vi "_sp3.vi"(5 "sp_data":T3={"total data num(1-3)"=2, "file_name"="", "SAVE OFF/ON"=TRUE, "ATT1"=5.0, "ATT2"=7.0, "SNAdatafile ATT1"=path "C:/Documents and Settings/?澤佳?/デスクトップ/MIX99/100217_ifbox/5dB.prn", "SNAdatafile ATT2"=path "C:/Documents and Settings/?澤佳?/デスクトップ/MIX99/100217_ifbox/7dB.prn", "ATTcal"=TRUE, "SP_set"={"start(GHz)"=3.5, "stop(GHz) "=12.5, "BW(MHz)"=8.0, "VBW(Hz)"=30.0, "ref(dBm)"=-45.0, "log(dB)"=1.0, "AVEG"=1, "AVEG ON/OFF"=FALSE, "Auto Align ON/OFF"=FALSE, "GPIB"="18", "point"=801}, "HOT/COLD"=0} {"HOT/COLD" items=["Manual", "Motor auto", "SIS V", "P0/P1", "sinlge data"]}, 6 "Control":T2={"GPIB_ATT"="28", "6501Dev#"=1, "GPIB_SP"="18", "GPIB_PM"="13", "GPIB_DSA"="11", "GPIB_DMM (TPD)"="23", "GPIB_MPI"="2", "mortor設定"=[{"Axis"=0, "ID"=0, "HIspeed"=200.0, "LOspeed"=100.0, "ACCEL(ms)"=100.0, "Sratio"=50.0, "フリーラン\n"=TRUE, "文字列"="DSB HOT/COLD"}, {"Axis"=1, "ID"=0, "HIspeed"=4.0, "LOspeed"=4.0, "ACCEL(ms)"=100.0, "Sratio"=50.0, "フリーラン\n"=TRUE, "文字列"="SubMM Att"}], "DATAパス"=path "Z:/band10/Labview_ALMA/MIX95/test", "DBパス "=path "Z:/band10/Labview_ALMA/MIX95/test", "comment"="P1_Tmin", "ColdCarts"="003601", "Th"=295.0, "Tc"=77.0, "Set_SIS_volt"=2.1, "Offset"=0.0, "control"=0, "FreqLO"=800.0, "Set_Mag_Cur"=800.0, "MPI offset(mm)"=22.99, "HOT/COLD"=0} {"HOT/COLD" items=["DSB", "SBR", "GainComp"]; "control" items=["CLOSE LOOP", "OPEN LOOP", "Not Control"]}, 7 "Bias_LO_equip":T1={"Node address"=19, "CAN Interface"="CAN0", "Cartridge band"=10, "Slave Node in"={"Address"=19, "Serial Number"=[16, 71, 55, 76, 1, 8, 0, -15]}, "ObjHandle out"=170917952, "POL"=1, "sb"=1, "GPIB_SM (SIS S,V)"="24", "GPIB_DMM (SIS I)"="22", "GPIB_SM (MAG I) "="25", "GPIB_SG(LO)"="19", "GPIB_PW (PAMP) "="6", "GPIB_TMP1(8ch)"="12", "GPIB_TMP2(2ch)  "="13", "WCA_avg"=10, "Rsen"=10.0, "BiasModule"=1, "LOModule "=5, "WCA_LO_FREQ_SET"={"YTO Low freq. [GHz]"=14.42, "YTO High freq. [GHz]"=17.7, "Kvco"=1, "Lock Pol."=0, "SET LO FREQ"=97.111115, "Multiplier"=6.0, "YTO (HEX)"=2196, "YTO ( FREQ)"=16.178946, "NULL PLL INTEGRATOR"=FALSE}, "Res for"=0} {"Res for" items=["none", "series res", "parallel res"]; "WCA_LO_FREQ_SET"."YTO ( FREQ)" min=25 max=150 step=0.0001 format="%.3f"; "WCA_LO_FREQ_SET"."Multiplier" min=3 max=6 step=3; "WCA_LO_FREQ_SET"."SET LO FREQ" min=25 max=150 step=0.0001 format="%.3f"; "WCA_LO_FREQ_SET"."Lock Pol." items=["Lower", "Upper"]; "WCA_LO_FREQ_SET"."Kvco" items=["7.5MHz/V", "15MHz/V"]; "WCA_LO_FREQ_SET"."YTO High freq. [GHz]" format="%.3f"; "WCA_LO_FREQ_SET"."YTO Low freq. [GHz]" format="%.3f"; "LOModule" items=["Manual Gunn+PAMP"=0, "PLL GUNN+PAMP"=5, "B10Lab LO"=1, "WCA LO"=2, ""=3, "YIG発信器"=4, "none"=99]; "BiasModule" items=["B10Lab Bias"=0, "WCA BiasModule"=1, "none"=99]; "Slave Node in"."Serial Number" format="%.0x"; "Slave Node in"."Address" format="%.0x"; "Cartridge band" max=10 step=1; "Node address" format="%.0x"}) -> ()   [LabVIEW 2017]
uses:
  <vilib>/Utility/file.llb/Read From Spreadsheet File (DBL).vi
  <vilib>/express/express arith-compare/Formula/XNode/ExpressFormulaBlockNode.xnode
  <vilib>/gmath/NI_Gmath.lvlib
panel:
  in  "HOT/COLD AUTO":bool=TRUE
  in  "タブ制御器":enum32{"ページ 1", "ページ 2"}(tab)
  out "XYグラフ":cluster{dbl, dbl}[](graph)=[{3.5, -71.954}, {3.51125, -71.842}, {3.5225, -71.893}, {3.53375, -72.314}, {3.545, -72.393}, {3.55625, -71.859}, {3.5675, -71.184}, {3.57875, -69.995}, {3.59, -68.081}, {3.60125, -65.91}, {3.6125, -64.753}, {3.62375, -64.752}, {3.635, -65.026}, {3.64625, -65.45}, {3.6575, -64.906}, {3.66875, -63.764}, {3.68, -62.097}, {3.69125, -60.126}, {3.7025, -58.665}, {3.71375, -58.024}, {3.725, -57.93}, {3.73625, -57.927}, {3.7475, -57.979}, {3.75875, -57.611}, {3.77, -56.352}, {3.78125, -54.399}, {3.7925, -52.484}, {3.80375, -51.209}, {3.815, -50.629}, {3.82625, -50.38}, {3.8375, -50.206}, {3.84875, -50.084}, {3.86, -49.915}, {3.87125, -49.525}, {3.8825, -49.077}, {3.89375, -48.4}, {3.905, -47.812}, {3.91625, -47.508}, {3.9275, -47.326}, {3.93875, -47.27}, {3.95, -47.088}, {3.96125, -46.924}, {3.9725, -46.838}, {3.98375, -46.867}, {3.995, -46.862}, {4.00625, -46.788}, {4.0175, -46.715}, {4.02875, -46.722}, {4.04, -46.709}, {4.05125, -46.62}, {4.0625, -46.617}, {4.07375, -46.606}, {4.085, -46.621}, {4.09625, -46.532}, {4.1075, -46.451}, {4.11875, -46.457}, {4.13, -46.365}, {4.14125, -46.296}, {4.1525, -46.289}, {4.16375, -46.373}, {4.175, -46.372}, {4.18625, -46.286}, {4.1975, -46.224}, {4.20875, -46.246}, {4.22, -46.278}, {4.23125, -46.252}, {4.2425, -46.205}, {4.25375, -46.184}, {4.265, -46.167}, {4.27625, -46.168}, {4.2875, -46.147}, {4.29875, -46.094}, {4.31, -46.092}, {4.32125, -46.151}, {4.3325, -46.218}, {4.34375, -46.256}, {4.355, -46.233}, {4.36625, -46.182}, {4.3775, -46.22}, {4.38875, -46.223}, {4.4, -46.301}, {4.41125, -46.386}, {4.4225, -46.511}, {4.43375, -46.483}, {4.445, -46.367}, {4.45625, -46.279}, {4.4675, -46.251}, {4.47875, -46.241}, {4.49, -46.238}, {4.50125, -46.231}, {4.5125, -46.219}, {4.52375, -46.147}, {4.535, -46.095}, {4.54625, -46.112}, {4.5575, -46.151}, {4.56875, -46.067}, {4.58, -46.01}, {4.59125, -45.981}, {4.6025, -46.006}, {4.61375, -46.047}, {4.625, -46.085}, {4.63625, -46.099}, {4.6475, -46.104}, {4.65875, -46.087}, {4.67, -46.069}, {4.68125, -46.087}, {4.6925, -46.163}, {4.70375, -46.198}, {4.715, -46.218}, {4.72625, -46.189}, {4.7375, -46.188}, {4.74875, -46.232}, {4.76, -46.248}, {4.77125, -46.379}, {4.7825, -46.515}, {4.79375, -46.613}, {4.805, -46.671}, {4.81625, -46.713}, {4.8275, -46.773}, {4.83875, -46.799}, {4.85, -46.868}, {4.86125, -46.939}, {4.8725, -46.989}, {4.88375, -47.123}, {4.895, -47.176}, {4.90625, -47.133}, {4.9175, -47.123}, {4.92875, -47.067}, {4.94, -47.068}, {4.95125, -47.108}, {4.9625, -47.197}, {4.97375, -47.251}, {4.985, -47.163}, {4.99625, -47.078}, {5.0075, -47.106}, {5.01875, -47.261}, {5.03, -47.236}, {5.04125, -47.088}, {5.0525, -47.01}, {5.06375, -47.036}, {5.075, -47.175}, {5.08625, -47.19}, {5.0975, -47.053}, {5.10875, -46.876}, {5.12, -46.702}, {5.13125, -46.717}, {5.1425, -46.72}, {5.15375, -46.718}, {5.165, -46.753}, {5.17625, -46.853}, {5.1875, -46.973}, {5.19875, -47.25}, {5.21, -47.402}, {5.22125, -47.146}, {5.2325, -47.002}, {5.24375, -46.974}, {5.255, -46.975}, {5.26625, -47.063}, {5.2775, -47.135}, {5.28875, -47.209}, {5.3, -47.278}, {5.31125, -47.27}, {5.3225, -47.272}, {5.33375, -47.282}, {5.345, -47.266}, {5.35625, -47.26}, {5.3675, -47.263}, {5.37875, -47.404}, {5.39, -47.446}, {5.40125, -47.366}, {5.4125, -47.323}, {5.42375, -47.361}, {5.435, -47.465}, {5.44625, -47.472}, {5.4575, -47.381}, {5.46875, -47.304}, {5.48, -47.288}, {5.49125, -47.333}, {5.5025, -47.467}, {5.51375, -47.458}, {5.525, -47.323}, {5.53625, -47.264}, {5.5475, -47.27}, {5.55875, -47.335}, {5.57, -47.249}, {5.58125, -47.105}, {5.5925, -47.044}, {5.60375, -47.03}, {5.615, -47.109}, {5.62625, -47.09}, {5.6375, -46.967}, {5.64875, -46.926}, {5.66, -46.942}, {5.67125, -47.103}, {5.6825, -47.225}, {5.69375, -47.112}, {5.705, -46.983}, {5.71625, -46.925}, {5.7275, -46.934}, {5.73875, -46.981}, {5.75, -47.024}, {5.76125, -47.033}, {5.7725, -47.114}, {5.78375, -47.206}, {5.795, -47.097}, {5.80625, -47.025}, {5.8175, -46.985}, {5.82875, -46.993}, {5.84, -47.125}, {5.85125, -47.259}, {5.8625, -47.344}, {5.87375, -47.276}, {5.885, -47.267}, {5.89625, -47.347}, {5.9075, -47.507}, {5.91875, -47.473}, {5.93, -47.345}, {5.94125, -47.275}, {5.9525, -47.288}, {5.96375, -47.47}, {5.975, -47.534}, {5.98625, -47.542}, {5.9975, -47.499}, {6.00875, -47.515}, {6.02, -47.607}, {6.03125, -47.748}, {6.0425, -47.648}, {6.05375, -47.578}, {6.065, -47.508}, {6.07625, -47.476}, {6.0875, -47.547}, {6.09875, -47.594}, {6.11, -47.534}, {6.12125, -47.453}, {6.1325, -47.326}, {6.14375, -47.297}, {6.155, -47.288}, {6.16625, -47.203}, {6.1775, -47.151}, {6.18875, -47.076}, {6.2, -47.058}, {6.21125, -46.98}, {6.2225, -46.939}, {6.23375, -46.893}, {6.245, -46.988}, {6.25625, -47.016}, {6.2675, -46.998}, {6.27875, -46.991}, {6.29, -46.946}, {6.30125, -46.945}, {6.3125, -47.01}, {6.32375, -47.183}, {6.335, -47.328}, {6.34625, -47.41}, {6.3575, -47.315}, {6.36875, -47.32}, {6.38, -47.479}, {6.39125, -47.474}, {6.4025, -47.433}, {6.41375, -47.457}, {6.425, -47.6}, {6.43625, -47.833}, {6.4475, -47.912}, {6.45875, -47.849}, {6.47, -47.844}, {6.48125, -47.87}, {6.4925, -47.94}, {6.50375, -47.984}, {6.515, -47.973}, {6.52625, -47.994}, {6.5375, -48.059}, {6.54875, -48.054}, {6.56, -48.117}, {6.57125, -48.268}, {6.5825, -48.212}, {6.59375, -48.119}, {6.605, -48.06}, {6.61625, -48.022}, {6.6275, -47.989}, {6.63875, -47.931}, {6.65, -47.939}, {6.66125, -47.992}, {6.6725, -47.963}, {6.68375, -47.893}, {6.695, -47.572}, {6.70625, -47.495}, {6.7175, -47.442}, {6.72875, -47.459}, {6.74, -47.385}, {6.75125, -47.361}, {6.7625, -47.311}, {6.77375, -47.208}, {6.785, -47.211}, {6.79625, -47.241}, {6.8075, -47.208}, {6.81875, -47.2}, {6.83, -47.225}, {6.84125, -47.271}, {6.8525, -47.437}, {6.86375, -47.61}, {6.875, -47.614}, {6.88625, -47.644}, {6.8975, -47.731}, {6.90875, -47.757}, {6.92, -47.789}, {6.93125, -47.736}, {6.9425, -47.737}, {6.95375, -47.619}, {6.965, -47.373}, {6.97625, -47.303}, {6.9875, -47.287}, {6.99875, -47.276}, {7.01, -47.34}, {7.02125, -47.491}, {7.0325, -47.621}, {7.04375, -47.843}, {7.055, -47.873}, {7.06625, -47.802}, {7.0775, -47.764}, {7.08875, -47.787}, {7.1, -47.793}, {7.11125, -47.733}, {7.1225, -47.469}, {7.13375, -47.271}, {7.145, -47.145}, {7.15625, -47.097}, {7.1675, -47.072}, {7.17875, -47.143}, {7.19, -47.234}, {7.20125, -47.288}, {7.2125, -47.346}, {7.22375, -47.39}, {7.235, -47.533}, {7.24625, -47.358}, {7.2575, -47.209}, {7.26875, -47.056}, {7.28, -46.933}, {7.29125, -46.892}, {7.3025, -46.642}, {7.31375, -46.487}, {7.325, -46.441}, {7.33625, -46.415}, {7.3475, -46.343}, {7.35875, -46.318}, {7.37, -46.302}, {7.38125, -46.537}, {7.3925, -46.847}, {7.40375, -46.854}, {7.415, -46.841}, {7.42625, -46.902}, {7.4375, -47.021}, {7.44875, -47.161}, {7.46, -47.435}, {7.47125, -47.781}, {7.4825, -47.531}, {7.49375, -47.405}, {7.505, -47.501}, {7.51625, -47.665}, {7.5275, -47.625}, {7.53875, -47.527}, {7.55, -47.453}, {7.56125, -47.592}, {7.5725, -47.723}, {7.58375, -47.43}, {7.595, -47.291}, {7.60625, -47.215}, {7.6175, -47.141}, {7.62875, -47.18}, {7.64, -47.309}, {7.65125, -47.525}, {7.6625, -47.415}, {7.67375, -47.178}, {7.685, -47.025}, {7.69625, -47.063}, {7.7075, -47.163}, {7.71875, -47.172}, {7.73, -47.341}, {7.74125, -47.497}, {7.7525, -47.465}, {7.76375, -47.238}, {7.775, -47.125}, {7.78625, -47.038}, {7.7975, -47.035}, {7.80875, -46.956}, {7.82, -46.887}, {7.83125, -46.691}, {7.8425, -46.535}, {7.85375, -46.453}, {7.865, -46.413}, {7.87625, -46.469}, {7.8875, -46.594}, {7.89875, -46.746}, {7.91, -46.859}, {7.92125, -47.036}, {7.9325, -47.214}, {7.94375, -47.294}, {7.955, -47.195}, {7.96625, -47.173}, {7.9775, -47.245}, {7.98875, -47.48}, {8.0, -47.468}, {8.01125, -47.138}, {8.0225, -46.85}, {8.03375, -46.737}, {8.045, -46.672}, {8.05625, -46.651}, {8.0675, -46.728}, {8.07875, -46.881}, {8.09, -47.039}, {8.10125, -47.059}, {8.1125, -47.027}, {8.12375, -47.041}, {8.135, -47.131}, {8.14625, -47.264}, {8.1575, -47.113}, {8.16875, -46.901}, {8.18, -46.669}, {8.19125, -46.499}, {8.2025, -46.442}, {8.21375, -46.451}, {8.225, -46.571}, {8.23625, -46.545}, {8.2475, -46.48}, {8.25875, -46.493}, {8.27, -46.494}, {8.28125, -46.454}, {8.2925, -46.493}, {8.30375, -46.766}, {8.315, -46.888}, {8.32625, -46.929}, {8.3375, -46.778}, {8.34875, -46.53}, {8.36, -46.506}, {8.37125, -46.633}, {8.3825, -46.912}, {8.39375, -47.149}, {8.405, -47.02}, {8.41625, -47.011}, {8.4275, -47.041}, {8.43875, -46.9}, {8.45, -46.848}, {8.46125, -46.941}, {8.4725, -47.126}, {8.48375, -47.289}, {8.495, -47.597}, {8.50625, -47.67}, {8.5175, -47.639}, {8.52875, -47.57}, {8.54, -47.643}, {8.55125, -47.999}, {8.5625, -48.482}, {8.57375, -48.445}, {8.585, -48.386}, {8.59625, -48.295}, {8.6075, -48.254}, {8.61875, -48.367}, {8.63, -48.398}, {8.64125, -48.483}, {8.6525, -48.862}, {8.66375, -48.682}, {8.675, -48.434}, {8.68625, -48.456}, {8.6975, -48.453}, {8.70875, -48.478}, {8.72, -48.475}, {8.73125, -48.559}, {8.7425, -48.753}, {8.75375, -48.633}, {8.765, -48.485}, {8.77625, -48.4}, {8.7875, -48.376}, {8.79875, -48.436}, {8.81, -48.56}, {8.82125, -48.668}, {8.8325, -48.756}, {8.84375, -48.81}, {8.855, -48.76}, {8.86625, -48.771}, {8.8775, -48.915}, {8.88875, -48.911}, {8.9, -48.871}, {8.91125, -48.87}, {8.9225, -48.91}, {8.93375, -48.989}, {8.945, -48.962}, {8.95625, -49.024}, {8.9675, -49.068}, {8.97875, -49.178}, {8.99, -49.307}, {9.00125, -49.438}, {9.0125, -49.343}, {9.02375, -49.306}, {9.035, -49.359}, {9.04625, -49.633}, {9.0575, -49.932}, {9.06875, -49.957}, {9.08, -49.924}, {9.09125, -49.955}, {9.1025, -50.016}, {9.11375, -50.034}, {9.125, -50.167}, {9.13625, -50.212}, {9.1475, -50.193}, {9.15875, -50.317}, {9.17, -50.568}, {9.18125, -50.694}, {9.1925, -50.942}, {9.20375, -50.843}, {9.215, -50.756}, {9.22625, -50.768}, {9.2375, -50.987}, {9.24875, -50.892}, {9.26, -50.838}, {9.27125, -50.868}, {9.2825, -50.777}, {9.29375, -50.499}, {9.305, -50.274}, {9.31625, -50.154}, {9.3275, -50.137}, {9.33875, -50.183}, {9.35, -50.199}, {9.36125, -50.095}, {9.3725, -50.004}, {9.38375, -49.996}, {9.395, -50.088}, {9.40625, -50.265}, {9.4175, -50.351}, {9.42875, -50.126}, {9.44, -49.893}, {9.45125, -49.901}, {9.4625, -49.87}, {9.47375, -49.79}, {9.485, -49.584}, {9.49625, -49.419}, {9.5075, -49.492}, {9.51875, -49.658}, {9.53, -49.972}, {9.54125, -50.161}, {9.5525, -50.298}, {9.56375, -50.405}, {9.575, -50.455}, {9.58625, -50.619}, {9.5975, -50.83}, {9.60875, -51.11}, {9.62, -51.061}, {9.63125, -51.029}, {9.6425, -51.011}, {9.65375, -51.013}, {9.665, -51.056}, {9.67625, -51.14}, {9.6875, -51.281}, {9.69875, -51.296}, {9.71, -51.39}, {9.72125, -51.515}, {9.7325, -51.685}, {9.74375, -51.81}, {9.755, -51.972}, {9.76625, -52.069}, {9.7775, -52.084}, {9.78875, -52.083}, {9.8, -52.012}, {9.81125, -52.005}, {9.8225, -51.769}, {9.83375, -51.503}, {9.845, -51.371}, {9.85625, -51.273}, {9.8675, -51.381}, {9.87875, -51.376}, {9.89, -51.116}, {9.90125, -50.863}, {9.9125, -50.64}, {9.92375, -50.582}, {9.935, -50.576}, {9.94625, -50.736}, {9.9575, -50.904}, {9.96875, -50.964}, {9.98, -51.343}, {9.99125, -51.665}, {10.0025, -51.61}, {10.01375, -51.443}, {10.025, -51.439}, {10.03625, -51.317}, {10.0475, -51.287}, {10.05875, -51.528}, {10.07, -51.818}, {10.08125, -51.83}, {10.0925, -51.847}, {10.10375, -51.65}, {10.115, -51.395}, {10.12625, -51.146}, {10.1375, -51.112}, {10.14875, -51.144}, {10.16, -51.204}, {10.17125, -51.391}, {10.1825, -51.63}, {10.19375, -51.824}, {10.205, -51.848}, {10.21625, -51.941}, {10.2275, -52.093}, {10.23875, -52.046}, {10.25, -52.017}, {10.26125, -52.211}, {10.2725, -52.345}, {10.28375, -52.094}, {10.295, -51.887}, {10.30625, -51.816}, {10.3175, -51.905}, {10.32875, -52.242}, {10.34, -52.607}, {10.35125, -52.478}, {10.3625, -52.33}, {10.37375, -52.199}, {10.385, -52.036}, {10.39625, -52.019}, {10.4075, -52.159}, {10.41875, -52.303}, {10.43, -51.947}, {10.44125, -51.68}, {10.4525, -51.689}, {10.46375, -52.1}, {10.475, -52.598}, {10.48625, -52.325}, {10.4975, -52.164}, {10.50875, -52.263}, {10.52, -52.392}, {10.53125, -52.562}, {10.5425, -52.581}, {10.55375, -52.684}, {10.565, -52.683}, {10.57625, -52.908}, {10.5875, -53.461}, {10.59875, -54.026}, {10.61, -53.447}, {10.62125, -53.018}, {10.6325, -52.82}, {10.64375, -52.542}, {10.655, -52.227}, {10.66625, -51.967}, {10.6775, -51.823}, {10.68875, -51.83}, {10.7, -52.037}, {10.71125, -52.406}, {10.7225, -52.612}, {10.73375, -52.958}, {10.745, -53.193}, {10.75625, -53.38}, {10.7675, -53.503}, {10.77875, -53.482}, {10.79, -53.314}, {10.80125, -53.149}, {10.8125, -53.048}, {10.82375, -52.998}, {10.835, -53.048}, {10.84625, -53.039}, {10.8575, -53.25}, {10.86875, -53.51}, {10.88, -53.135}, {10.89125, -52.842}, {10.9025, -52.76}, {10.91375, -52.749}, {10.925, -53.082}, {10.93625, -53.424}, {10.9475, -53.489}, {10.95875, -53.431}, {10.97, -53.218}, {10.98125, -53.083}, {10.9925, -52.862}, {11.00375, -52.702}, {11.015, -52.589}, {11.02625, -52.395}, {11.0375, -52.351}, {11.04875, -52.493}, {11.06, -52.789}, {11.07125, -52.657}, {11.0825, -52.484}, {11.09375, -52.469}, {11.105, -52.515}, {11.11625, -52.733}, {11.1275, -52.718}, {11.13875, -52.712}, {11.15, -52.705}, {11.16125, -52.773}, {11.1725, -52.926}, {11.18375, -53.285}, {11.195, -53.63}, {11.20625, -53.688}, {11.2175, -53.507}, {11.22875, -53.483}, {11.24, -53.567}, {11.25125, -53.872}, {11.2625, -53.942}, {11.27375, -53.909}, {11.285, -53.962}, {11.29625, -54.009}, {11.3075, -54.13}, {11.31875, -54.282}, {11.33, -54.512}, {11.34125, -54.993}, {11.3525, -54.907}, {11.36375, -54.589}, {11.375, -54.365}, {11.38625, -54.0}, {11.3975, -53.84}, {11.40875, -53.788}, {11.42, -53.787}, {11.43125, -53.917}, {11.4425, -54.185}, {11.45375, -54.528}, {11.465, -54.871}, {11.47625, -54.573}, {11.4875, -54.388}, {11.49875, -54.433}, {11.51, -54.668}, {11.52125, -54.887}, {11.5325, -55.037}, {11.54375, -55.076}, {11.555, -55.133}, {11.56625, -54.956}, {11.5775, -54.649}, {11.58875, -54.536}, {11.6, -54.508}, {11.61125, -54.439}, {11.6225, -54.513}, {11.63375, -54.746}, {11.645, -55.053}, {11.65625, -55.34}, {11.6675, -55.542}, {11.67875, -55.519}, {11.69, -55.354}, {11.70125, -55.181}, {11.7125, -55.089}, {11.72375, -54.965}, {11.735, -54.856}, {11.74625, -54.901}, {11.7575, -55.157}, {11.76875, -55.323}, {11.78, -55.286}, {11.79125, -55.066}, {11.8025, -54.962}, {11.81375, -54.984}, {11.825, -55.109}, {11.83625, -55.261}, {11.8475, -55.068}, {11.85875, -54.862}, {11.87, -54.783}, {11.88125, -54.818}, {11.8925, -54.664}, {11.90375, -54.832}, {11.915, -54.974}, {11.92625, -55.083}, {11.9375, -55.33}, {11.94875, -55.714}, {11.96, -56.097}, {11.97125, -55.931}, {11.9825, -55.862}, {11.99375, -55.928}, {12.005, -56.047}, {12.01625, -55.985}, {12.0275, -55.847}, {12.03875, -56.034}, {12.05, -55.922}, {12.06125, -55.8}, {12.0725, -55.771}, {12.08375, -55.593}, {12.095, -55.6}, {12.10625, -55.918}, {12.1175, -56.305}, {12.12875, -56.413}, {12.14, -56.4}, {12.15125, -56.827}, {12.1625, -57.471}, {12.17375, -58.045}, {12.185, -57.987}, {12.19625, -57.899}, {12.2075, -57.938}, {12.21875, -57.8}, {12.23, -58.004}, {12.24125, -58.753}, {12.2525, -59.581}, {12.26375, -60.009}, {12.275, -59.706}, {12.28625, -59.607}, {12.2975, -59.689}, {12.30875, -60.204}, {12.32, -61.1}, {12.33125, -62.589}, {12.3425, -64.312}, {12.35375, -65.705}, {12.365, -66.003}, {12.37625, -65.213}, {12.3875, -64.672}, {12.39875, -64.666}, {12.41, -64.945}, {12.42125, -65.677}, {12.4325, -66.563}, {12.44375, -67.347}, {12.455, -67.766}, {12.46625, -67.937}, {12.4775, -68.115}, {12.48875, -68.108}, {12.5, -67.876}]
  out "XYグラフ 2":cluster{dbl, dbl}[](graph)=[{3.5, 262.8761923486348}, {3.51125, 265.3941119007726}, {3.5225, 261.20275301828303}, {3.53375, 254.61452613630323}, {3.545, 265.256944327723}, {3.55625, 256.71770445279355}, {3.5675, 253.29895702347693}, {3.57875, 255.931422963521}, {3.59, 257.1114683734254}, {3.60125, 255.75498871941952}, {3.6125, 250.5281702924347}, {3.62375, 240.4459191545401}, {3.635, 245.18716604138476}, {3.64625, 238.9567024993202}, {3.6575, 236.97953138656834}, {3.66875, 254.50165799946515}, {3.68, 242.07864861705457}, {3.69125, 244.50359101739548}, {3.7025, 224.949128515961}, {3.71375, 225.85065303629233}, {3.725, 228.89158214555707}, {3.73625, 229.3093007737749}, {3.7475, 228.17456602724567}, {3.75875, 231.41887343795008}, {3.77, 240.36727143390723}, {3.78125, 224.65040280568107}, {3.7925, 227.2627743063754}, {3.80375, 239.43391314174212}, {3.815, 247.8165740086698}, {3.82625, 245.15636147038293}, {3.8375, 240.82133483850794}, {3.84875, 244.21563567548085}, {3.86, 244.4827666625702}, {3.87125, 244.08831190861994}, {3.8825, 241.8090904197592}, {3.89375, 244.34243732142812}, {3.905, 244.67617340165324}, {3.91625, 242.69332978130743}, {3.9275, 240.47841129027896}, {3.93875, 235.47071382602226}, {3.95, 241.93528131929722}, {3.96125, 241.89546730654737}, {3.9725, 241.86385478544392}, {3.98375, 236.56768322757807}, {3.995, 238.7902448928445}, {4.00625, 247.50639151841088}, {4.0175, 245.57315502756728}, {4.02875, 241.90119061580842}, {4.04, 243.33931405889274}, {4.05125, 243.10170518604278}, {4.0625, 244.04149874278417}, {4.07375, 246.9641892769639}, {4.085, 238.61123449304475}, {4.09625, 242.9462880124439}, {4.1075, 244.5051542938281}, {4.11875, 244.12106797294564}, {4.13, 240.57466833749857}, {4.14125, 240.8274300472488}, {4.1525, 243.30389434626068}, {4.16375, 240.68284134010386}, {4.175, 239.34447201355923}, {4.18625, 245.05443426912723}, {4.1975, 245.682449223128}, {4.20875, 245.80306076988367}, {4.22, 248.0206300592133}, {4.23125, 242.02207084394269}, {4.2425, 246.9183927125329}, {4.25375, 243.05566615613813}, {4.265, 249.08045120777058}, {4.27625, 247.13970788273744}, {4.2875, 240.30192904146838}, {4.29875, 245.41878418214426}, {4.31, 241.7558889355493}, {4.32125, 241.31125347787935}, {4.3325, 243.2220561500085}, {4.34375, 231.30252460707732}, {4.355, 235.44495546231832}, {4.36625, 244.56412835893218}, {4.3775, 237.0241031165103}, {4.38875, 239.04193968622735}, {4.4, 236.43738406649962}, {4.41125, 236.94651077829408}, {4.4225, 234.76613596800598}, {4.43375, 236.369466168867}, {4.445, 236.8802182641571}, {4.45625, 239.50967040948262}, {4.4675, 237.3156198339352}, {4.47875, 233.35482141391896}, {4.49, 234.39853864941963}, {4.50125, 232.93326616359997}, {4.5125, 230.8352049801077}, {4.52375, 235.480258435589}, {4.535, 238.0804283666065}, {4.54625, 243.96822176961183}, {4.5575, 233.56300311786632}, {4.56875, 237.6484876135124}, {4.58, 237.07719132394985}, {4.59125, 240.06151036000696}, {4.6025, 239.16401930247414}, {4.61375, 240.853494620256}, {4.625, 237.24016928691904}, {4.63625, 237.0012418390217}, {4.6475, 236.19054957073072}, {4.65875, 232.79019526262627}, {4.67, 234.41802454613145}, {4.68125, 236.71013995490105}, {4.6925, 234.94960077269158}, {4.70375, 242.74225771843138}, {4.715, 230.69626423612328}, {4.72625, 237.99671249942847}, {4.7375, 243.19972698657756}, {4.74875, 241.78564535897496}, {4.76, 246.68989579012796}, {4.77125, 233.77252393131778}, {4.7825, 232.74807333114165}, {4.79375, 237.3375087150141}, {4.805, 236.843220223869}, {4.81625, 238.62876135740984}, {4.8275, 237.65852913341678}, {4.83875, 242.60928819707286}, {4.85, 236.5923218121674}, {4.86125, 233.1555591792413}, {4.8725, 248.21294191750152}, {4.88375, 238.63927518318636}, {4.895, 236.6411303958895}, {4.90625, 238.84550812970093}, {4.9175, 239.8289353237909}, {4.92875, 233.29071763362768}, {4.94, 232.47060195525304}, {4.95125, 233.54853283996468}, {4.9625, 232.80149118225611}, {4.97375, 234.11503048456947}, {4.985, 234.4759190982286}, {4.99625, 236.5417413984665}, {5.0075, 237.41562271675028}, {5.01875, 239.9997205474734}, {5.03, 238.58613987506754}, {5.04125, 232.48363592932222}, {5.0525, 235.53513669533723}, {5.06375, 234.33804621510708}, {5.075, 241.269198219873}, {5.08625, 234.02323477825186}, {5.0975, 242.29718074124258}, {5.10875, 236.02463840576507}, {5.12, 236.95944040804943}, {5.13125, 238.55613692219285}, {5.1425, 242.4470435889024}, {5.15375, 239.3502543997521}, {5.165, 238.91000188022844}, {5.17625, 239.31305101575524}, {5.1875, 237.61117258685775}, {5.19875, 231.08459955814823}, {5.21, 233.77715027839795}, {5.22125, 237.3641274054419}, {5.2325, 240.43558006862244}, {5.24375, 238.64482239024633}, {5.255, 237.84575437419429}, {5.26625, 229.46983026008294}, {5.2775, 231.8887895591687}, {5.28875, 231.4694475478289}, {5.3, 237.29809610715094}, {5.31125, 234.7988368263242}, {5.3225, 231.60295499583188}, {5.33375, 231.44738786408712}, {5.345, 231.0886709663173}, {5.35625, 232.24037455797222}, {5.3675, 241.48036100089934}, {5.37875, 239.14444206738256}, {5.39, 232.69403961963692}, {5.40125, 228.888336281852}, {5.4125, 234.86172420860981}, {5.42375, 243.2137160998339}, {5.435, 238.10850425624025}, {5.44625, 238.01391341341093}, {5.4575, 244.4606049467267}, {5.46875, 235.9959874073434}, {5.48, 235.66977533038096}, {5.49125, 241.22113266632343}, {5.5025, 235.4424424452742}, {5.51375, 234.75165758630135}, {5.525, 236.904921957093}, {5.53625, 233.19135361535803}, {5.5475, 238.73861462072895}, {5.55875, 234.362693329857}, {5.57, 231.1092409249881}, {5.58125, 240.97681653730191}, {5.5925, 236.11047643013305}, {5.60375, 238.8333518067794}, {5.615, 234.80131919923548}, {5.62625, 240.5471271966678}, {5.6375, 245.2831523438754}, {5.64875, 240.4902315241231}, {5.66, 237.9620851683432}, {5.67125, 230.4328301720102}, {5.6825, 239.50182239080038}, {5.69375, 234.4162930352756}, {5.705, 234.0895207836703}, {5.71625, 240.33606037010668}, {5.7275, 236.6216409093753}, {5.73875, 238.91798976099656}, {5.75, 240.45256994610926}, {5.76125, 241.58658612417847}, {5.7725, 240.64394879499338}, {5.78375, 239.6687587740024}, {5.795, 236.78517017888439}, {5.80625, 244.71226767073722}, {5.8175, 242.07287083691554}, {5.82875, 240.6671952503448}, {5.84, 239.75129069739876}, {5.85125, 242.84880690337437}, {5.8625, 244.14384194504845}, {5.87375, 251.51335341434242}, {5.885, 243.2387154019542}, {5.89625, 242.08147342549773}, {5.9075, 238.7540532528154}, {5.91875, 243.6630214289088}, {5.93, 245.04777609947007}, {5.94125, 233.21307186732122}, {5.9525, 236.2713141317444}, {5.96375, 238.75123820734723}, {5.975, 232.45486514265716}, {5.98625, 233.1525875454649}, {5.9975, 234.47642078491666}, {6.00875, 235.21148113842006}, {6.02, 231.35071654999257}, {6.03125, 233.37148508457844}, {6.0425, 237.17292627401238}, {6.05375, 235.96291980952483}, {6.065, 238.4998630658882}, {6.07625, 239.33592227187125}, {6.0875, 239.56943294171472}, {6.09875, 245.68912636163802}, {6.11, 239.9855888097656}, {6.12125, 238.6005209798928}, {6.1325, 244.43366773104208}, {6.14375, 239.38084164181677}, {6.155, 240.51500824164705}, {6.16625, 248.3078400032811}, {6.1775, 244.54928015200326}, {6.18875, 244.891538238819}, {6.2, 234.9028179015556}, {6.21125, 244.33720219255375}, {6.2225, 239.93746573150216}, {6.23375, 244.3345437782873}, {6.245, 235.76493507964028}, {6.25625, 236.50270646691186}, {6.2675, 239.53997300690804}, {6.27875, 240.5210503745131}, {6.29, 242.6904342917291}, {6.30125, 241.85719495206573}, {6.3125, 239.21305219088632}, {6.32375, 240.95980458159138}, {6.335, 245.11569869908118}, {6.34625, 235.30020702565508}, {6.3575, 236.62832317521605}, {6.36875, 242.63255486024457}, {6.38, 241.07463321439533}, {6.39125, 238.64498885564035}, {6.4025, 240.8370961374533}, {6.41375, 250.48291734875818}, {6.425, 242.23010056126168}, {6.43625, 241.86313805650508}, {6.4475, 242.5339414927508}, {6.45875, 244.06245324447366}, {6.47, 242.48403386240577}, {6.48125, 245.21096794973263}, {6.4925, 239.56236431315028}, {6.50375, 240.5088590943489}, {6.515, 242.56318295195382}, {6.52625, 243.2441109619106}, {6.5375, 235.59976596646771}, {6.54875, 238.32045913099856}, {6.56, 232.18702961090986}, {6.57125, 235.277709121525}, {6.5825, 231.17244472135286}, {6.59375, 232.61300692594648}, {6.605, 234.9907912634667}, {6.61625, 233.2564761170557}, {6.6275, 235.46629793802603}, {6.63875, 240.60339705851462}, {6.65, 235.5114294836484}, {6.66125, 233.62810982507642}, {6.6725, 245.54352552564856}, {6.68375, 239.7081078826325}, {6.695, 238.69356266733556}, {6.70625, 237.93953819852965}, {6.7175, 240.9883827058091}, {6.72875, 241.62665404519646}, {6.74, 241.6478200251123}, {6.75125, 239.49712326867018}, {6.7625, 236.62575183297074}, {6.77375, 239.0779488557507}, {6.785, 232.2937306632569}, {6.79625, 241.26692445446858}, {6.8075, 241.55295568738504}, {6.81875, 239.13799275922133}, {6.83, 236.03059739864116}, {6.84125, 236.67546695019885}, {6.8525, 239.29192223310244}, {6.86375, 232.47697648679082}, {6.875, 236.72593299486232}, {6.88625, 235.54392932908488}, {6.8975, 232.9215804711459}, {6.90875, 234.40025095245593}, {6.92, 234.93811941053224}, {6.93125, 235.90666263395394}, {6.9425, 233.23040255411934}, {6.95375, 236.07409801220228}, {6.965, 236.20293118503076}, {6.97625, 234.23397717468362}, {6.9875, 234.01507133689316}, {6.99875, 237.64451228286822}, {7.01, 237.4902969130223}, {7.02125, 230.8142640160615}, {7.0325, 234.16973815774838}, {7.04375, 231.64730153553384}, {7.055, 233.71451171706772}, {7.06625, 228.9855316623015}, {7.0775, 235.75703262057172}, {7.08875, 231.5401184496277}, {7.1, 230.66008129722263}, {7.11125, 223.36780769764633}, {7.1225, 231.1573002100412}, {7.13375, 231.3069442304926}, {7.145, 232.7306246963992}, {7.15625, 226.9077729737077}, {7.1675, 235.23308226670454}, {7.17875, 236.25867213581648}, {7.19, 234.04116468076853}, {7.20125, 233.02538370774073}, {7.2125, 235.74539656076809}, {7.22375, 240.2126163114857}, {7.235, 231.36624203818386}, {7.24625, 233.87182651249896}, {7.2575, 242.36520208398622}, {7.26875, 243.66967319058415}, {7.28, 240.45223241868135}, {7.29125, 238.69201710897974}, {7.3025, 245.23654600085968}, {7.31375, 240.16942273294234}, {7.325, 233.65913306732105}, {7.33625, 237.4351143740074}, {7.3475, 239.88078222578528}, {7.35875, 232.59677595567882}, {7.37, 237.09695710259012}, {7.38125, 226.16369761214264}, {7.3925, 228.1864955101728}, {7.40375, 230.00521062815062}, {7.415, 227.47173310934394}, {7.42625, 232.39804239338903}, {7.4375, 230.59332719738467}, {7.44875, 231.60223376076019}, {7.46, 240.82888806093496}, {7.47125, 234.03686200232752}, {7.4825, 234.98284594051054}, {7.49375, 239.11954211626002}, {7.505, 234.60827004465327}, {7.51625, 236.97799974980555}, {7.5275, 242.62238821253285}, {7.53875, 239.77628304411172}, {7.55, 238.60568420653144}, {7.56125, 242.64790598751338}, {7.5725, 232.32141170457018}, {7.58375, 222.29663010445483}, {7.595, 232.03149113271076}, {7.60625, 231.49892227184748}, {7.6175, 238.48168131480875}, {7.62875, 238.33894263285455}, {7.64, 233.01128265051528}, {7.65125, 233.56951272117226}, {7.6625, 237.74376421684474}, {7.67375, 240.6769415467833}, {7.685, 233.82393048277135}, {7.69625, 232.758299698207}, {7.7075, 230.17961814309942}, {7.71875, 234.2099287347315}, {7.73, 227.36808415706992}, {7.74125, 230.3022351057765}, {7.7525, 230.42650259457005}, {7.76375, 230.76230782966724}, {7.775, 232.7883992193337}, {7.78625, 230.0114693817353}, {7.7975, 226.43722137063833}, {7.80875, 234.07087596250915}, {7.82, 232.52623233214618}, {7.83125, 235.97868804062747}, {7.8425, 235.4469622889499}, {7.85375, 234.86358325591786}, {7.865, 228.06914859486395}, {7.87625, 232.62594435332386}, {7.8875, 227.5696233177269}, {7.89875, 235.82947420871204}, {7.91, 241.10142457464283}, {7.92125, 238.4441263314762}, {7.9325, 233.56249652164814}, {7.94375, 237.88535348009378}, {7.955, 236.02254309492622}, {7.96625, 235.85764690354944}, {7.9775, 233.0661469050419}, {7.98875, 233.19272132627682}, {8.0, 235.85551603623927}, {8.01125, 230.09626222180023}, {8.0225, 237.62261162535884}, {8.03375, 236.84544300145743}, {8.045, 233.67527800204567}, {8.05625, 234.27551437502913}, {8.0675, 233.7286337590969}, {8.07875, 229.5997025866425}, {8.09, 227.23423691019087}, {8.10125, 228.47230880739676}, {8.1125, 227.86271962619202}, {8.12375, 232.463605488288}, {8.135, 234.30635037065102}, {8.14625, 229.6060847787881}, {8.1575, 225.64980741052537}, {8.16875, 224.0812265944788}, {8.18, 222.97766048632343}, {8.19125, 228.3284068357738}, {8.2025, 223.1692976092905}, {8.21375, 229.12868694498533}, {8.225, 221.51875250354183}, {8.23625, 226.45991880536397}, {8.2475, 227.43540173378133}, {8.25875, 227.9723639607012}, {8.27, 232.29612454341665}, {8.28125, 237.4992153213221}, {8.2925, 243.4930016807316}, {8.30375, 238.2353484602185}, {8.315, 241.43704058953614}, {8.32625, 238.42700629312}, {8.3375, 235.88137629459905}, {8.34875, 246.21978139201144}, {8.36, 244.16967509822203}, {8.37125, 236.61442228183583}, {8.3825, 229.4699789829297}, {8.39375, 233.72487000473765}, {8.405, 237.83106534460183}, {8.41625, 231.46124082172528}, {8.4275, 228.51136671976812}, {8.43875, 229.45690327503593}, {8.45, 222.52729325146515}, {8.46125, 220.87718191202873}, {8.4725, 218.59471872319602}, {8.48375, 219.71122077260281}, {8.495, 219.91018635585093}, {8.50625, 220.80302977432342}, {8.5175, 221.33871976853712}, {8.52875, 227.7544629840319}, {8.54, 232.9602081243155}, {8.55125, 224.7500358304345}, {8.5625, 227.48990784524185}, {8.57375, 232.90999856246725}, {8.585, 232.89887003213332}, {8.59625, 227.68305746110354}, {8.6075, 232.53779305318113}, {8.61875, 233.00294007665403}, {8.63, 228.04363626408292}, {8.64125, 236.4272780533551}, {8.6525, 232.21806352488161}, {8.66375, 230.61418867146708}, {8.675, 229.02333985518464}, {8.68625, 231.47861181234308}, {8.6975, 239.03306482746154}, {8.70875, 232.98545153851953}, {8.72, 233.82694089682298}, {8.73125, 232.43497302918655}, {8.7425, 231.22206804234173}, {8.75375, 234.38288652749125}, {8.765, 233.35674920324948}, {8.77625, 234.59154803122354}, {8.7875, 234.87452736492185}, {8.79875, 236.73453019845516}, {8.81, 226.0064035364036}, {8.82125, 232.58829515107007}, {8.8325, 226.52994617511945}, {8.84375, 228.04435821637733}, {8.855, 232.3146698237139}, {8.86625, 231.53785168896553}, {8.8775, 227.07873290165648}, {8.88875, 232.8579521241822}, {8.9, 227.83176357720086}, {8.91125, 229.2329759013122}, {8.9225, 232.92552402805853}, {8.93375, 229.88657438958376}, {8.945, 237.9632935400163}, {8.95625, 229.71770843841622}, {8.9675, 233.28786796684392}, {8.97875, 238.262251795725}, {8.99, 236.25699242534742}, {9.00125, 223.79800974155782}, {9.0125, 227.7459089646673}, {9.02375, 233.50948939937405}, {9.035, 232.05740443703579}, {9.04625, 231.13749918776114}, {9.0575, 229.29816591664553}, {9.06875, 230.70510349950396}, {9.08, 228.6025630488676}, {9.09125, 226.84275969331517}, {9.1025, 230.46179423454356}, {9.11375, 232.15266952365374}, {9.125, 236.80077845955478}, {9.13625, 230.5344759713846}, {9.1475, 228.2254984502071}, {9.15875, 228.14715419053087}, {9.17, 223.7159104233841}, {9.18125, 231.1457462549388}, {9.1925, 222.4265545342947}, {9.20375, 224.6329733121259}, {9.215, 227.05692636223557}, {9.22625, 221.80237428208747}, {9.2375, 209.46074220323055}, {9.24875, 222.2412978961111}, {9.26, 220.67737348551353}, {9.27125, 215.9010466673391}, {9.2825, 225.8209257229435}, {9.29375, 218.32665273388068}, {9.305, 222.46578864082656}, {9.31625, 220.46850832792373}, {9.3275, 228.64202028848953}, {9.33875, 225.61803055979397}, {9.35, 221.36349809661706}, {9.36125, 220.49490893965805}, {9.3725, 230.71332970810323}, {9.38375, 236.12779217851786}, {9.395, 239.1492148535695}, {9.40625, 235.90767740573435}, {9.4175, 214.61665805492456}, {9.42875, 225.96104861210353}, {9.44, 233.92425626351513}, {9.45125, 232.51642300578075}, {9.4625, 240.29112194011296}, {9.47375, 234.91971428786343}, {9.485, 242.62761160512716}, {9.49625, 241.28493839691882}, {9.5075, 232.99498041127976}, {9.51875, 239.0467123190332}, {9.53, 233.2554857213408}, {9.54125, 228.75673549432722}, {9.5525, 228.17652787617644}, {9.56375, 229.4133494121902}, {9.575, 234.46214525473616}, {9.58625, 232.48837113562234}, {9.5975, 226.9435143501272}, {9.60875, 221.718824844387}, {9.62, 219.51227150565296}, {9.63125, 217.29460627019327}, {9.6425, 232.1579155970462}, {9.65375, 223.62031446941495}, {9.665, 222.67862569782235}, {9.67625, 233.69958026537208}, {9.6875, 232.6472130009311}, {9.69875, 231.2805530366355}, {9.71, 234.8862213754746}, {9.72125, 239.2762352699338}, {9.7325, 233.58755911696798}, {9.74375, 237.4397505764616}, {9.755, 227.84796320387392}, {9.76625, 232.2221575836937}, {9.7775, 240.8157854555772}, {9.78875, 232.26474453020413}, {9.8, 230.02031577831073}, {9.81125, 228.5285567286357}, {9.8225, 231.82868748140365}, {9.83375, 226.4452562833874}, {9.845, 222.49457390799947}, {9.85625, 225.75120731489147}, {9.8675, 228.72424536783635}, {9.87875, 223.4869258639065}, {9.89, 232.92201010850044}, {9.90125, 232.34414609400045}, {9.9125, 236.03940115207533}, {9.92375, 226.80822756877552}, {9.935, 226.3920653483931}, {9.94625, 234.95112605630447}, {9.9575, 224.04600711848317}, {9.96875, 233.16417997717426}, {9.98, 232.32780812380918}, {9.99125, 226.81217898795092}, {10.0025, 224.83348013600187}, {10.01375, 230.3577070612578}, {10.025, 228.628451453206}, {10.03625, 229.2238998758718}, {10.0475, 231.2071287236024}, {10.05875, 231.97743156442678}, {10.07, 220.96825255362825}, {10.08125, 227.7663836879507}, {10.0925, 224.9530240249836}, {10.10375, 224.1549459971992}, {10.115, 227.5771966487341}, {10.12625, 235.63713278752414}, {10.1375, 230.99156320365282}, {10.14875, 229.03005172273092}, {10.16, 231.5630228391997}, {10.17125, 232.3630392551307}, {10.1825, 230.97323682084104}, {10.19375, 225.71809579722353}, {10.205, 231.53968855543133}, {10.21625, 228.5379150295213}, {10.2275, 225.16924521114197}, {10.23875, 227.10834179876576}, {10.25, 229.78325147337267}, {10.26125, 223.37058624629125}, {10.2725, 220.03680845570108}, {10.28375, 209.8788851458008}, {10.295, 215.6732255118866}, {10.30625, 212.92089174318042}, {10.3175, 222.87850133162394}, {10.32875, 218.48616095198312}, {10.34, 216.06021505180797}, {10.35125, 217.9063627304262}, {10.3625, 214.47485586846503}, {10.37375, 220.12197770074573}, {10.385, 228.20315712157162}, {10.39625, 226.70264611460127}, {10.4075, 221.12333979738048}, {10.41875, 219.89351934249473}, {10.43, 221.19670255509038}, {10.44125, 221.58630903234442}, {10.4525, 219.25182222922922}, {10.46375, 219.9690261078238}, {10.475, 211.2978971038437}, {10.48625, 209.52691356593508}, {10.4975, 213.4114092600905}, {10.50875, 219.04007538796017}, {10.52, 222.50637189541638}, {10.53125, 213.51193969544872}, {10.5425, 222.8094346817436}, {10.55375, 228.68716505660208}, {10.565, 226.14109170819665}, {10.57625, 238.77423282051026}, {10.5875, 236.10032497295924}, {10.59875, 229.72938587905023}, {10.61, 230.16388988045034}, {10.62125, 228.99402525673872}, {10.6325, 229.29161089644808}, {10.64375, 227.57546759288394}, {10.655, 225.10374434909085}, {10.66625, 221.48916936174857}, {10.6775, 224.27033644630853}, {10.68875, 218.43093854477195}, {10.7, 224.7442015144185}, {10.71125, 222.0825323893974}, {10.7225, 217.59896060505872}, {10.73375, 219.9113330739886}, {10.745, 228.1575983370558}, {10.75625, 229.7851866879694}, {10.7675, 230.85662873641874}, {10.77875, 232.40259534748748}, {10.79, 229.99778921565107}, {10.80125, 222.1697019367816}, {10.8125, 225.2204675526488}, {10.82375, 229.66143845259293}, {10.835, 222.13383894091396}, {10.84625, 221.98341961791576}, {10.8575, 221.9242973915478}, {10.86875, 217.81712987829812}, {10.88, 219.22926482040862}, {10.89125, 220.14042301997293}, {10.9025, 226.6567215820497}, {10.91375, 223.43380141425234}, {10.925, 226.77800688591185}, {10.93625, 221.5999888060867}, {10.9475, 232.3857075085164}, {10.95875, 229.08725247082705}, {10.97, 231.05778456275638}, {10.98125, 234.44742521251595}, {10.9925, 235.67417668666857}, {11.00375, 222.78545686872002}, {11.015, 227.81354448631933}, {11.02625, 223.33411323462408}, {11.0375, 231.16646586696643}, {11.04875, 225.53380253148933}, {11.06, 231.66341266827033}, {11.07125, 229.521914597968}, {11.0825, 224.3311463884755}, {11.09375, 222.22379818533997}, {11.105, 224.7836035626071}, {11.11625, 216.10971381666667}, {11.1275, 225.35100782215946}, {11.13875, 217.95978704623252}, {11.15, 222.26761631155102}, {11.16125, 225.24141426849644}, {11.1725, 221.6705745917931}, {11.18375, 230.55981667086218}, {11.195, 228.26188609323154}, {11.20625, 219.85077495988725}, {11.2175, 225.3302832894331}, {11.22875, 226.3013449459716}, {11.24, 230.15399556283907}, {11.25125, 223.75786512987145}, {11.2625, 232.71123360794863}, {11.27375, 233.35669688289232}, {11.285, 221.2554915765746}, {11.29625, 233.30895525396113}, {11.3075, 225.92143501167885}, {11.31875, 221.5140583241589}, {11.33, 230.0738345347478}, {11.34125, 226.32132042269473}, {11.3525, 234.4894933433795}, {11.36375, 231.7880397039943}, {11.375, 229.02944166183389}, {11.38625, 239.54319113258478}, {11.3975, 232.7416664178743}, {11.40875, 228.96026054402887}, {11.42, 233.55680833785533}, {11.43125, 242.38846252753075}, {11.4425, 226.27917876248472}, {11.45375, 228.22382351481974}, {11.465, 230.15699028098467}, {11.47625, 234.1687046742876}, {11.4875, 235.98345633693322}, {11.49875, 232.01170905855264}, {11.51, 216.27046236437945}, {11.52125, 233.50808745838074}, {11.5325, 228.03002315876483}, {11.54375, 231.186635898348}, {11.555, 229.36652484496923}, {11.56625, 229.83969922981547}, {11.5775, 234.4411262664677}, {11.58875, 233.16414726364806}, {11.6, 232.90371386781715}, {11.61125, 234.56326899491413}, {11.6225, 236.20533475938055}, {11.63375, 232.82631933967852}, {11.645, 235.55393932753006}, {11.65625, 238.34119554511585}, {11.6675, 233.80254125862723}, {11.67875, 236.6905628092792}, {11.69, 244.20959660864307}, {11.70125, 232.199564278271}, {11.7125, 246.03244464818144}, {11.72375, 241.6994301936939}, {11.735, 239.415623924205}, {11.74625, 236.1673812810697}, {11.7575, 232.22410312285345}, {11.76875, 240.2830902781452}, {11.78, 243.34933520716984}, {11.79125, 240.28518523996314}, {11.8025, 230.94235533263387}, {11.81375, 230.00998020072845}, {11.825, 225.52844596330843}, {11.83625, 227.29714693811417}, {11.8475, 223.5269575641194}, {11.85875, 229.60787608278056}, {11.87, 223.0834171584205}, {11.88125, 217.03470640155606}, {11.8925, 217.35175410311797}, {11.90375, 218.80219775388335}, {11.915, 215.8469740139766}, {11.92625, 221.81711772159613}, {11.9375, 225.78022532062508}, {11.94875, 219.1372280966623}, {11.96, 223.141195940916}, {11.97125, 227.70347431240907}, {11.9825, 239.48514092595966}, {11.99375, 243.973293919654}, {12.005, 246.7173750187963}, {12.01625, 250.43809513536766}, {12.0275, 242.82797064796745}, {12.03875, 247.01873821027843}, {12.05, 255.5506105688013}, {12.06125, 242.03554037883825}, {12.0725, 240.91656035082735}, {12.08375, 240.4347282350332}, {12.095, 241.1999182855732}, {12.10625, 241.37754240325168}, {12.1175, 237.38024618055294}, {12.12875, 236.8473098909505}, {12.14, 235.9978581322268}, {12.15125, 234.8436938098652}, {12.1625, 233.12512881185557}, {12.17375, 232.79789133840345}, {12.185, 246.19643619682205}, {12.19625, 233.03381176627053}, {12.2075, 237.220330654482}, {12.21875, 227.66743295666166}, {12.23, 239.01126400961033}, {12.24125, 240.73786158188688}, {12.2525, 242.2057911392195}, {12.26375, 246.72635155835147}, {12.275, 236.4466159413481}, {12.28625, 239.50860311591057}, {12.2975, 242.31500961593247}, {12.30875, 241.81425773564004}, {12.32, 236.8990790941474}, {12.33125, 246.73756024154582}, {12.3425, 248.8837307453541}, {12.35375, 246.04819914506268}, {12.365, 247.28966942078188}, {12.37625, 249.54711316192234}, {12.3875, 249.3612221547051}, {12.39875, 243.4154361345046}, {12.41, 251.06398772639454}, {12.42125, 253.47507201630216}, {12.4325, 252.72189150157476}, {12.44375, 247.79329209195546}, {12.455, 246.85043142367306}, {12.46625, 250.9742969849379}, {12.4775, 247.74481543884627}, {12.48875, 239.17429212977498}, {12.5, 239.48179846468716}]
  out "wait":dbl=53.6186552
  in  "OKボタン":bool
  in  "スライド":i16(slide)=2 min=1 max=3 scale=1.0..2.0
  # "LO freq. [GHz]"
  # "YTO LOW\n/High Freq."
  # "ZERO Intgrtr"
  # "Node Address"
  # "Serial Number"
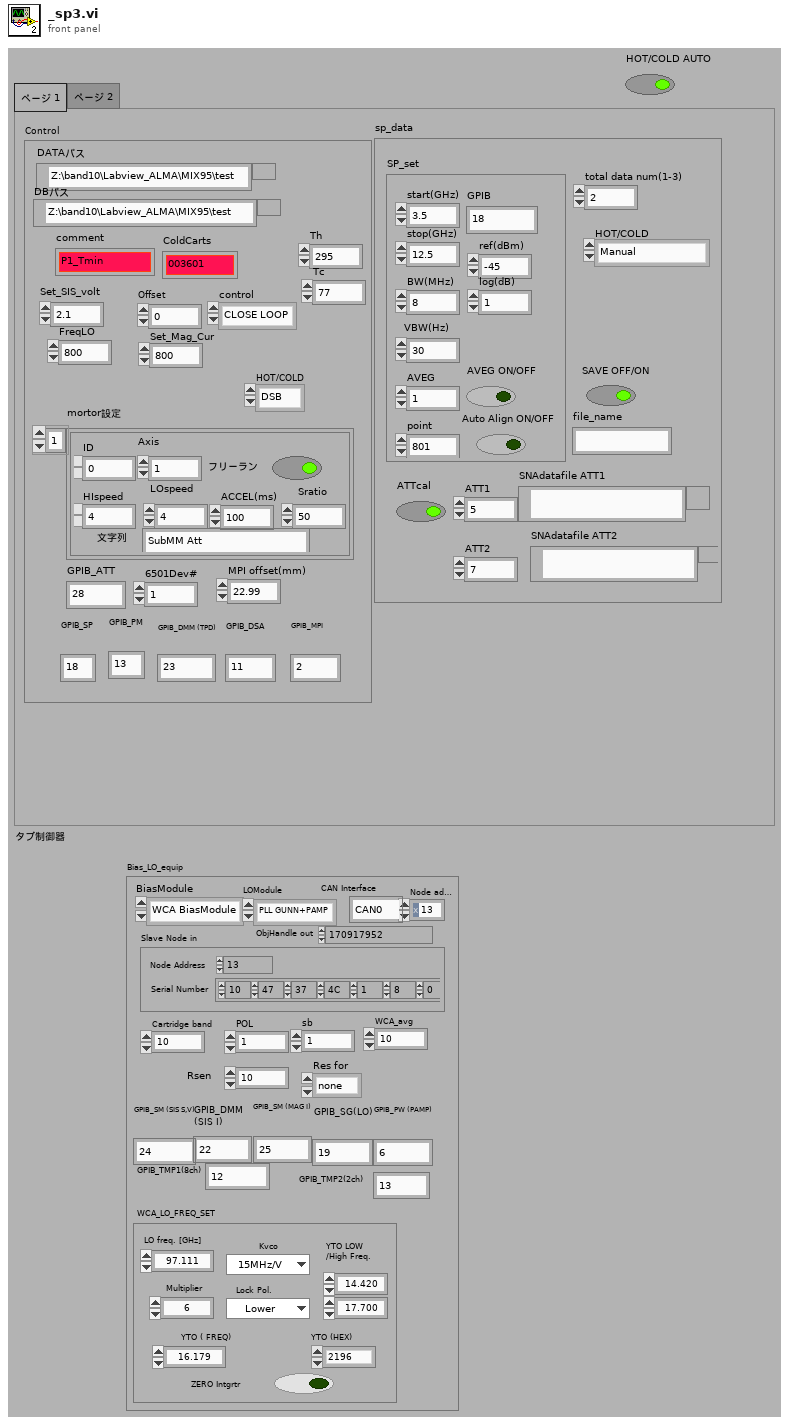
[diagram p1: front panel]
types:
  T1 = cluster{"Node address":u16, "CAN Interface":string, "Cartridge band":u32, "Slave Node in":cluster{"Address":i16, "Serial Number":i8[]}, "ObjHandle out":u32, "POL":u32, "sb":u32, "GPIB_SM (SIS S,V)":string, "GPIB_DMM (SIS I)":string, "GPIB_SM (MAG I) ":string, "GPIB_SG(LO)":string, "GPIB_PW (PAMP) ":string, "GPIB_TMP1(8ch)":string, "GPIB_TMP2(2ch)  ":string, "WCA_avg":i32, "Rsen":dbl, "BiasModule":u16, "LOModule ":u16, "WCA_LO_FREQ_SET":cluster{"YTO Low freq. [GHz]":sgl, "YTO High freq. [GHz]":sgl, "Kvco":u16, "Lock Pol.":u16, "SET LO FREQ":sgl, "Multiplier":sgl, "YTO (HEX)":u16, "YTO ( FREQ)":sgl, "NULL PLL INTEGRATOR":bool}, "Res for":u16}
  T2 = cluster{"GPIB_ATT":string, "6501Dev#":i16, "GPIB_SP":string, "GPIB_PM":string, "GPIB_DSA":string, "GPIB_DMM (TPD)":string, "GPIB_MPI":string, "mortor設定":cluster{"Axis":i16, "ID":i16, "HIspeed":dbl, "LOspeed":dbl, "ACCEL(ms)":dbl, "Sratio":dbl, "フリーラン\n":bool, "文字列":string}[], "DATAパス":path, "DBパス ":path, "comment":string, "ColdCarts":string, "Th":dbl, "Tc":dbl, "Set_SIS_volt":dbl, "Offset":dbl, "control":u16, "FreqLO":dbl, "Set_Mag_Cur":dbl, "MPI offset(mm)":dbl, "HOT/COLD":u16}
  T3 = cluster{"total data num(1-3)":i16, "file_name":string, "SAVE OFF/ON":bool, "ATT1":dbl, "ATT2":dbl, "SNAdatafile ATT1":path, "SNAdatafile ATT2":path, "ATTcal":bool, "SP_set":cluster{"start(GHz)":dbl, "stop(GHz) ":dbl, "BW(MHz)":dbl, "VBW(Hz)":dbl, "ref(dBm)":dbl, "log(dB)":dbl, "AVEG":i16, "AVEG ON/OFF":bool, "Auto Align ON/OFF":bool, "GPIB":string, "point":i16}, "HOT/COLD":u16}
  T4 = cluster{"start(GHz)":dbl, "stop(GHz) ":dbl, "BW(MHz)":dbl, "VBW(Hz)":dbl, "ref(dBm)":dbl, "log(dB)":dbl, "AVEG":i16, "AVEG ON/OFF":bool, "Auto Align ON/OFF":bool, "GPIB":string, "point":i16}
  T5 = cluster{"Axis":i16, "ID":i16, "HIspeed":dbl, "LOspeed":dbl, "ACCEL(ms)":dbl, "Sratio":dbl, "フリーラン\n":bool, "文字列":string}[]
  T6 = cluster{"Axis":i16, "ID":i16, "HIspeed":dbl, "LOspeed":dbl, "ACCEL(ms)":dbl, "Sratio":dbl, "フリーラン\n":bool, "文字列":string}
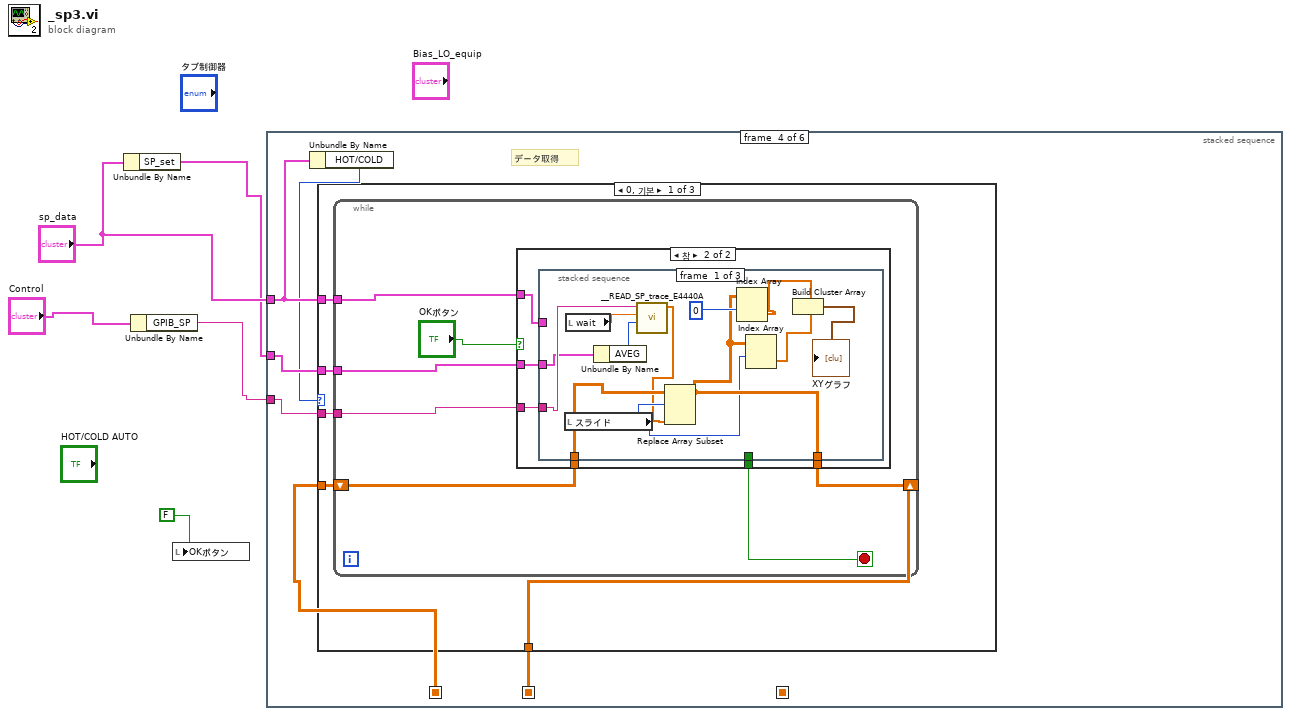
[diagram p0: block diagram]
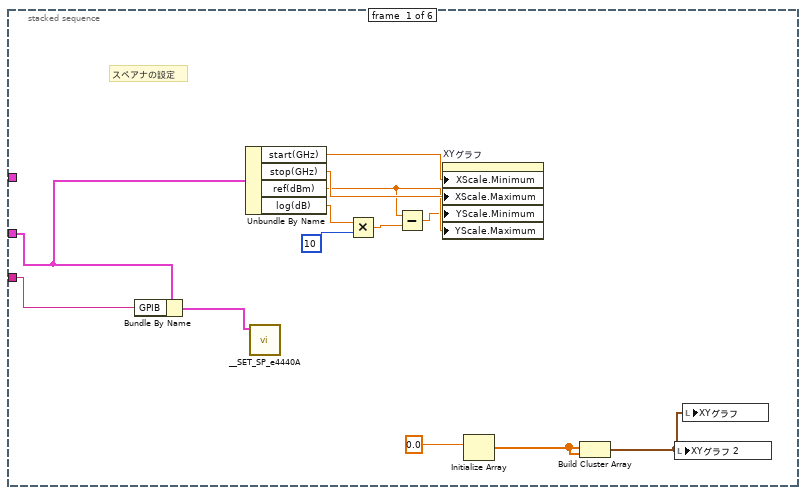
[diagram p2: hidden frame]
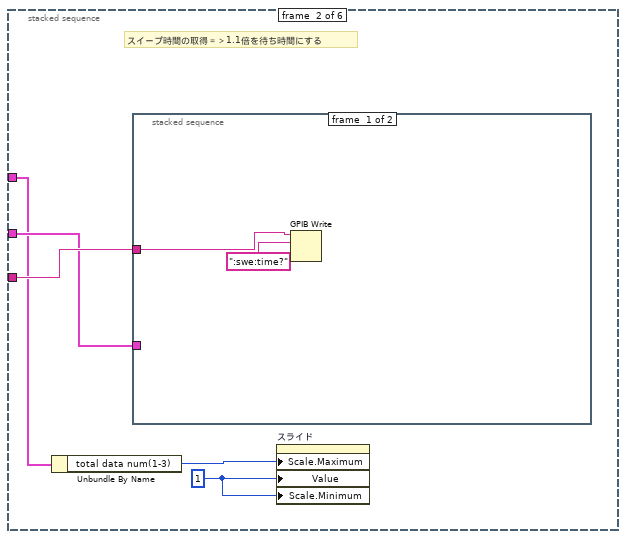
[diagram p3: hidden frame]
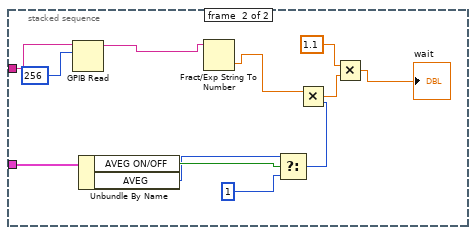
[diagram p4: hidden frame]
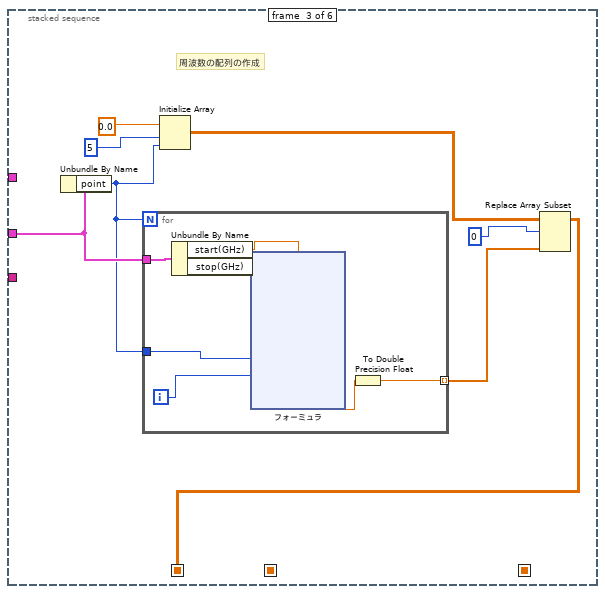
[diagram p5: hidden frame]
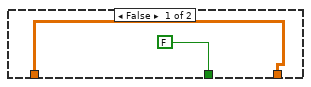
[diagram p6: hidden frame]
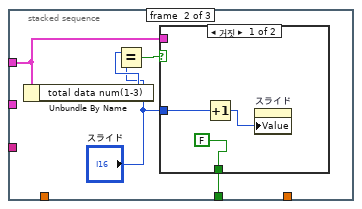
[diagram p7: hidden frame]
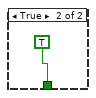
[diagram p8: hidden frame]
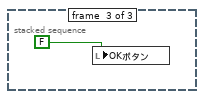
[diagram p9: hidden frame]
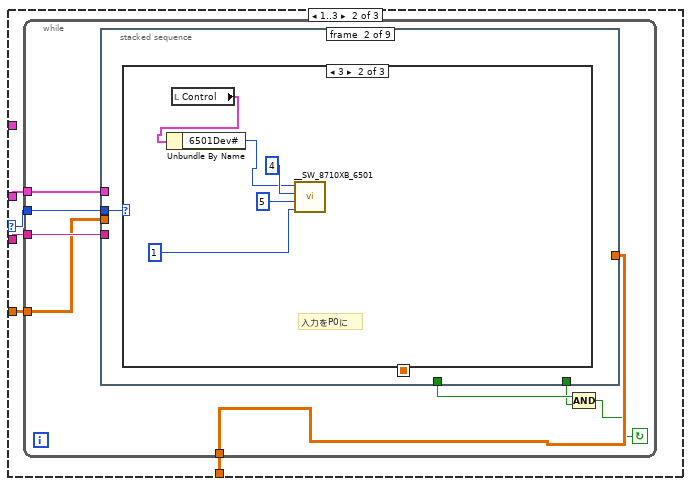
[diagram p10: hidden frame]
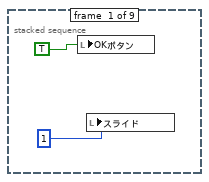
[diagram p11: hidden frame]
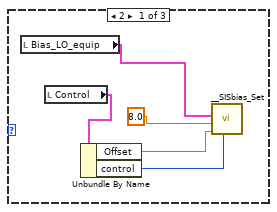
[diagram p12: hidden frame]
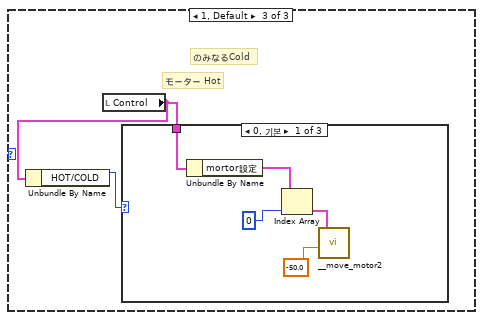
[diagram p13: hidden frame]
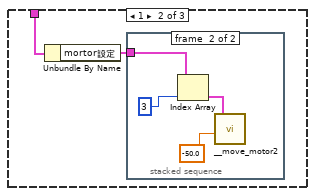
[diagram p14: hidden frame]
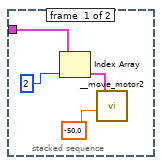
[diagram p15: hidden frame]
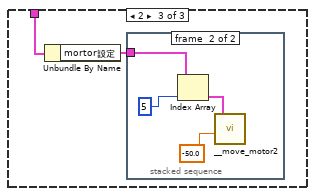
[diagram p16: hidden frame]
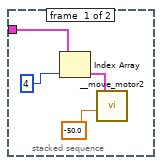
[diagram p17: hidden frame]
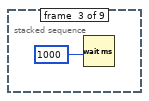
[diagram p18: hidden frame]
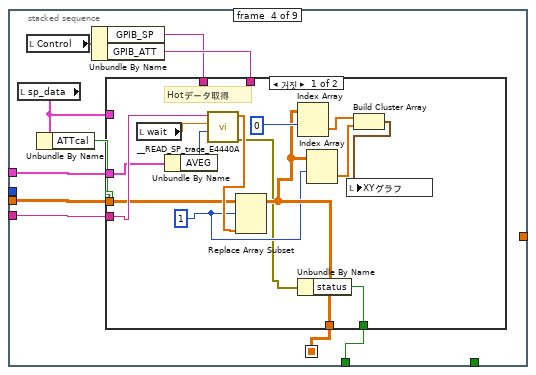
[diagram p19: hidden frame]
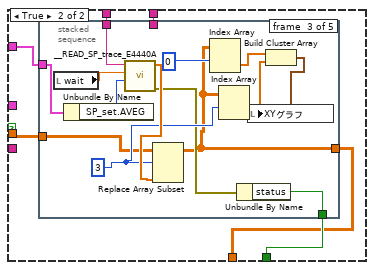
[diagram p20: hidden frame]
diagram:
  n1 = Unbundle By Name("sp_data") -> ("SP_set"=w3:T4)
  n2 = Unbundle By Name("Control") -> ("GPIB_SP"=w2:string)
  n3 = local write "OKボタン"(FALSE) -> ()
  n4 = stacked-sequence {
    seq-local: [_ _ w38 _ _ _] -> [_ _ _ w70 _ _]
    seq-local: [_ _ _ w69 _ _] -> [_ _ _ _ w357 _]
    seq-local: [_ _ _ _ w350 _] -> [_ _ _ _ _ w458]
    tunnel: w3 -> [w11 w22 w43 w72 w355 _]
    tunnel: w2 -> [w10 w23 _ w71 _ _]
    tunnel: "sp_data" -> [_ w21 _ w68 w356 w459]
    frame #0 {
      # "スペアナの設定"
      n5 = Bundle By Name(cluster=w11, "GPIB"=w10) -> (w9:T4)
      n6 = Unbundle By Name(w11) -> ("start(GHz)"=w18:dbl, "stop(GHz)"=w17:dbl, "ref(dBm)"=w15:dbl, "log(dB)"=w16:dbl)
      n7 = call "__SET_SP_e4440A.vi"("SP"=w9) -> ()  [unwired: 7 in]
      n8 = Multiply(x=w16, y=10) -> (x*y=w14:dbl)
      n9 = Subtract(x=w15, y=w14) -> (x-y=w13:dbl)
      n10 = property on="XYグラフ" class="XYGraph (决拜茄)"("XScale.Minimum"=w18, "XScale.Maximum"=w17, "YScale.Minimum"=w13, "YScale.Maximum"=w15) -> ()  [unwired: 2 in, 2 out]
      n11 = Initialize Array(0.0) -> (w7:dbl[])  [unwired: 1 in]
      n12 = Build Cluster Array(w7, w7) -> (w8:cluster{dbl, dbl}[])
      n13 = local write "XYグラフ 2"(w8) -> ()
      n14 = local write "XYグラフ"(w8) -> ()
    }
    frame #1 {
      w19 = 1
      # "スイープ時間の取得＝＞1.1倍を待ち時間にする"
      n15 = Unbundle By Name(w21) -> ("total data num(1-3)"=w20:i16)
      n16 = stacked-sequence {
        tunnel: w23 -> [w24 w35]
        tunnel: w22 -> [_ w34]
        frame #0 {
          n17 = GPIB Write(0:w24, 1:":swe:time?") -> ()  [unwired: 3 in, 2 out]
        }
        frame #1 {
          n18 = GPIB Read(0:w35, 1:256) -> (5:w36:string)  [unwired: 3 in, 2 out]
          n19 = Unbundle By Name(w34) -> ("AVEG ON/OFF"=w33:bool, "AVEG"=w32:i16)
          n20 = Fract/Exp String To Number(string=w36) -> (number=w29:dbl)  [unwired: 3 in, 1 out]
          n21 = Select(t=w32, s=w33, f=1) -> (s? t:f=w30:i32)
          n22 = Multiply(x=w29, y=w30) -> (x*y=w27:dbl)
          n23 = Multiply(x=1.1, y=w27) -> (x*y=→"wait":dbl)
        }
      }
      n24 = property on="スライド" class="Slide (决拜茄)"("Scale.Maximum"=w20, "Value"=w19, "Scale.Minimum"=w19) -> ()  [unwired: 2 in, 2 out]
    }
    frame #2 {
      # "周波数の配列の作成"
      n25 = Unbundle By Name(w43) -> ("point"=w42:i16)
      n26 = for {
        N: w42 -> [_]
        tunnel: w43 -> [w52]
        tunnel: w42 -> [w50]
        tunnel: [w46] -> w41 mode=indexing
        i -> [w51]
        n27 = Unbundle By Name(w52) -> ("start(GHz)"=w48:dbl, "stop(GHz)"=w49:dbl)
        n28 = xnode "フォーミュラ"("start"=w48, "stop"=w49, "point"=w50, "num"=w51) -> ("結果"=w47:dbl)  [unwired: 1 in, 1 out]
        n29 = To Double Precision Float(number=w47) -> (double precision float=w46:dbl)
      }
      n30 = Initialize Array(0.0, 5, w42) -> (w40:dbl[][])
      n31 = Replace Array Subset(array=w40, new element=w41, index (row)=0) -> (w38:dbl[][])  [unwired: 1 in]
    }
    frame #3 {
      # "データ取得"
      n32 = Unbundle By Name(w68) -> ("HOT/COLD"=w67:u16)
      n33 = case shown="0, 기본" w67 {
        selector: w67 -> [_ w115 w277]
        tunnel: w68 -> [w77 _ _]
        tunnel: w72 -> [w76 w118 w280]
        tunnel: w71 -> [w75 w119 w281]
        tunnel: w70 -> [w74 w117 w279]
        tunnel: [w73 w116 w278] -> w69
        frame 0, Default {
          n34 = while {
            tunnel: w77 -> [w82]
            tunnel: w76 -> [w84]
            tunnel: w75 -> [w83]
            shift-right: [w78] -> w73
            shift-left: w74 -> [w79]
            stop <- w81 stop-if-true
            n35 = case shown="참" "OKボタン" {
              tunnel: w84 -> [_ w92]
              tunnel: w83 -> [_ w91]
              tunnel: w82 -> [_ w90]
              tunnel: [FALSE w89] -> w81
              tunnel: w79 -> [w85 w88]
              tunnel: [w85 w87] -> w78
              frame False {
              }
              frame True {
                n36 = stacked-sequence {
                  tunnel: w92 -> [w94 _ _]
                  tunnel: w91 -> [w97 _ _]
                  tunnel: w90 -> [_ w106 _]
                  tunnel: [_ w107 _] -> w89
                  tunnel: w88 -> [w104 _ _]
                  tunnel: [w102 _ _] -> w87
                  frame #0 {
                    n37 = local read "スライド"() -> (w101:i16)
                    n38 = local read "wait"() -> (w96:dbl)
                    n39 = Unbundle By Name(w94) -> ("AVEG"=w93:i16)
                    n40 = call "__READ_SP_trace_E4440A.vi"("AVG(0-100)"=w93, "wait(s)"=w96, "GPIB"=w97) -> ("data"=w95:dbl[])  [unwired: 3 in, 1 out]
                    n41 = Replace Array Subset(array=w104, new element=w95, index (row)=w101) -> (w102:dbl[][])  [unwired: 1 in]
                    n42 = Index Array(array=w102, index (row)=0) -> (element=w100:dbl[])  [unwired: 1 in]
                    n43 = Index Array(array=w102, index (row)=w101) -> (element=w99:dbl[])  [unwired: 1 in]
                    n44 = Build Cluster Array(w100, w99) -> (→"XYグラフ":cluster{dbl, dbl}[])
                  }
                  frame #1 {
                    n45 = Unbundle By Name(w106) -> ("total data num(1-3)"=w109:i16)
                    n46 = Equal?(x=w109, y="スライド") -> (x = y?=w108:bool)
                    n47 = case shown="거짓" w108 {
                      tunnel: [FALSE TRUE] -> w107
                      tunnel: "スライド" -> [w112 _]
                      tunnel: w106 -> [_ _]
                      frame False {
                        n48 = Increment(x=w112) -> (x+1=w110:i16)
                        n49 = property on="スライド" class="Slide (决拜茄)"("Value"=w110) -> ()  [unwired: 2 in, 2 out]
                      }
                      frame True {
                      }
                    }
                  }
                  frame #2 {
                    n50 = local write "OKボタン"(FALSE) -> ()
                  }
                }
              }
            }
          }
        }
        frame 1..3 {
          n51 = while {
            tunnel: w119 -> [w127]
            tunnel: w118 -> [w126]
            tunnel: w117 -> [w125]
            tunnel: [w124] -> w116
            tunnel: w115 -> [w120]
            stop <- w123 continue-if-true
            n52 = stacked-sequence {
              seq-local: [_ _ _ w175 _ _ _ _ _] -> [_ _ _ _ _ _ _ w269 _]
              tunnel: w126 -> [_ _ _ w177 _ _ _ w271 _]
              tunnel: w127 -> [_ _ _ w178 _ _ _ w274 _]
              tunnel: w125 -> [_ _ _ w176 _ _ _ _ _]
              tunnel: [_ _ _ _ _ _ _ w261 _] -> w124
              tunnel: [_ _ _ w174 _ _ _ _ _] -> w122
              tunnel: [_ _ _ _ _ _ _ w262 _] -> w121
              tunnel: w120 -> [_ w130 _ _ w221 _ _ _ _]
              frame #0 {
                n53 = local write "OKボタン"(TRUE) -> ()
                n54 = local write "スライド"(1) -> ()
              }
              frame #1 {
                n55 = case shown="3" w130 {
                  frame 2 {
                    n56 = local read "Bias_LO_equip"() -> (w135:T1)
                    n57 = local read "Control"() -> (w134:T2)
                    n58 = Unbundle By Name(w134) -> ("Offset"=w132:dbl, "control"=w133:u16)
                    n59 = call "__SISbias_Set.vi"("SIS　Mode"=w133, "Offset"=w132, "Set_V"=8.0, "Bias_LO_equip"=w135) -> ()  [unwired: 7 in, 1 out]
                  }
                  frame 3 {
                    # "入力をP0に"
                    n60 = local read "Control"() -> (w138:T2)
                    n61 = Unbundle By Name(w138) -> ("6501Dev#"=w137:i16)
                    n62 = call "__SW_8710XB_6501.vi"("Path(1..6)"=1, "ch(1..6)"=5, "bit(4or6)"=4, "Dev(1,2..)"=w137) -> ()
                  }
                  frame 1, Default {
                    # "のみなるCold"
                    # "モーター Hot"
                    n63 = local read "Control"() -> (w142:T2)
                    n64 = Unbundle By Name(w142) -> ("HOT/COLD"=w141:u16)
                    n65 = case shown="0, 기본" w141 {
                      tunnel: w142 -> [w145 w149 w159]
                      frame 0, Default {
                        n66 = Unbundle By Name(w145) -> ("mortor設定"=w144:T5)
                        n67 = Index Array(array=w144, index=0) -> (element=w143:T6)
                        n68 = call "__move_motor2.vi"("Moving distance"=-50.0, "motor setup"=w143) -> ()  [unwired: 2 in, 2 out]
                      }
                      frame 1 {
                        n69 = Unbundle By Name(w149) -> ("mortor設定"=w148:T5)
                        n70 = stacked-sequence {
                          tunnel: w148 -> [w151 w155]
                          frame #0 {
                            n71 = Index Array(array=w151, index=2) -> (element=w150:T6)
                            n72 = call "__move_motor2.vi"("Moving distance"=-50.0, "motor setup"=w150) -> ()  [unwired: 2 in, 2 out]
                          }
                          frame #1 {
                            n73 = Index Array(array=w155, index=3) -> (element=w154:T6)
                            n74 = call "__move_motor2.vi"("Moving distance"=-50.0, "motor setup"=w154) -> ()  [unwired: 2 in, 2 out]
                          }
                        }
                      }
                      frame 2 {
                        n75 = Unbundle By Name(w159) -> ("mortor設定"=w158:T5)
                        n76 = stacked-sequence {
                          tunnel: w158 -> [w161 w165]
                          frame #0 {
                            n77 = Index Array(array=w161, index=4) -> (element=w160:T6)
                            n78 = call "__move_motor2.vi"("Moving distance"=-50.0, "motor setup"=w160) -> ()  [unwired: 2 in, 2 out]
                          }
                          frame #1 {
                            n79 = Index Array(array=w165, index=5) -> (element=w164:T6)
                            n80 = call "__move_motor2.vi"("Moving distance"=-50.0, "motor setup"=w164) -> ()  [unwired: 2 in, 2 out]
                          }
                        }
                      }
                    }
                  }
                }
              }
              frame #2 {
                n81 = Wait (ms)(milliseconds to wait=1000) -> ()  [unwired: 1 out]
              }
              frame #3 {
                n82 = local read "sp_data"() -> (w170:T3)
                n83 = local read "Control"() -> (w172:T2)
                n84 = Unbundle By Name(w170) -> ("ATTcal"=w173:bool)
                n85 = Unbundle By Name(w172) -> ("GPIB_SP"=w169:string, "GPIB_ATT"=w171:string)
                n86 = case shown="거짓" w173 {
                  tunnel: w178 -> [w192 _]
                  tunnel: w177 -> [w189 _]
                  tunnel: w176 -> [w187 w195]
                  tunnel: [w185 w193] -> w175
                  tunnel: [w179 w194] -> w174
                  tunnel: w171 -> [_ w198]
                  tunnel: w170 -> [_ w197]
                  tunnel: w169 -> [_ w196]
                  frame False {
                    w184 = 1
                    # "Hotデータ取得"
                    n87 = local read "wait"() -> (w191:dbl)
                    n88 = Unbundle By Name(w189) -> ("AVEG"=w188:i16)
                    n89 = call "__READ_SP_trace_E4440A.vi"("AVG(0-100)"=w188, "wait(s)"=w191, "GPIB"=w192) -> ("error out"=w180:errorcluster, "data"=w190:dbl[])  [unwired: 3 in]
                    n90 = Replace Array Subset(array=w187, new element=w190, index (row)=w184) -> (w185:dbl[][])  [unwired: 1 in]
                    n91 = Index Array(array=w185, index (row)=0) -> (element=w183:dbl[])  [unwired: 1 in]
                    n92 = Unbundle By Name(w180) -> ("status"=w179:bool)
                    n93 = Index Array(array=w185, index (row)=w184) -> (element=w182:dbl[])  [unwired: 1 in]
                    n94 = Build Cluster Array(w183, w182) -> (w181:cluster{dbl, dbl}[])
                    n95 = local write "XYグラフ"(w181) -> ()
                  }
                  frame True {
                    n96 = stacked-sequence {
                      tunnel: w197 -> [w200 _ w204 w217 _]
                      tunnel: [_ _ w207 _ _] -> w194
                      tunnel: [_ _ w206 _ _] -> w193
                      tunnel: w198 -> [w201 _ _ w219 _]
                      tunnel: w196 -> [_ _ w205 _ _]
                      tunnel: w195 -> [_ _ w203 _ _]
                      frame #0 {
                        n97 = Unbundle By Name(w200) -> ("ATT2"=w199:dbl)
                        n98 = call "__AttSet_11713A.vi"("ATT(dB)"=w199, "GPIB"=w201) -> ()  [unwired: 2 in]
                      }
                      frame #1 {
                        n99 = Wait (ms)(milliseconds to wait=1000) -> ()  [unwired: 1 out]
                      }
                      frame #2 {
                        w212 = 3
                        n100 = local read "wait"() -> (w216:dbl)
                        n101 = Unbundle By Name(w204) -> ("SP_set.AVEG"=w214:i16)
                        n102 = call "__READ_SP_trace_E4440A.vi"("AVG(0-100)"=w214, "wait(s)"=w216, "GPIB"=w205) -> ("error out"=w208:errorcluster, "data"=w215:dbl[])  [unwired: 3 in]
                        n103 = Replace Array Subset(array=w203, new element=w215, index (row)=w212) -> (w206:dbl[][])  [unwired: 1 in]
                        n104 = Index Array(array=w206, index (row)=0) -> (element=w211:dbl[])  [unwired: 1 in]
                        n105 = Index Array(array=w206, index (row)=w212) -> (element=w210:dbl[])  [unwired: 1 in]
                        n106 = Unbundle By Name(w208) -> ("status"=w207:bool)
                        n107 = Build Cluster Array(w211, w210) -> (w209:cluster{dbl, dbl}[])
                        n108 = local write "XYグラフ"(w209) -> ()
                      }
                      frame #3 {
                        n109 = Unbundle By Name(w217) -> ("ATT1"=w218:dbl)
                        n110 = call "__AttSet_11713A.vi"("ATT(dB)"=w218, "GPIB"=w219) -> ()  [unwired: 2 in]
                      }
                      frame #4 {
                        n111 = Wait (ms)(milliseconds to wait=1000) -> ()  [unwired: 1 out]
                      }
                    }
                  }
                }
              }
              frame #4 {
                # "モーター cold"
                n112 = case shown="2" w221 {
                  frame 1, Default {
                    n113 = local read "Control"() -> (w223:T2)
                    n114 = Unbundle By Name(w223) -> ("HOT/COLD"=w222:u16)
                    n115 = case shown="2" w222 {
                      tunnel: w223 -> [w226 w230 w240]
                      frame 0, Default {
                        n116 = Unbundle By Name(w226) -> ("mortor設定"=w225:T5)
                        n117 = Index Array(array=w225, index=0) -> (element=w224:T6)
                        n118 = call "__move_motor2.vi"("Moving distance"=50.0, "motor setup"=w224) -> ()  [unwired: 2 in, 2 out]
                      }
                      frame 1 {
                        n119 = Unbundle By Name(w230) -> ("mortor設定"=w229:T5)
                        n120 = stacked-sequence {
                          tunnel: w229 -> [w232 w236]
                          frame #0 {
                            n121 = Index Array(array=w232, index=2) -> (element=w231:T6)
                            n122 = call "__move_motor2.vi"("Moving distance"=50.0, "motor setup"=w231) -> ()  [unwired: 2 in, 2 out]
                          }
                          frame #1 {
                            n123 = Index Array(array=w236, index=3) -> (element=w235:T6)
                            n124 = call "__move_motor2.vi"("Moving distance"=50.0, "motor setup"=w235) -> ()  [unwired: 2 in, 2 out]
                          }
                        }
                      }
                      frame 2 {
                        n125 = Unbundle By Name(w240) -> ("mortor設定"=w239:T5)
                        n126 = stacked-sequence {
                          tunnel: w239 -> [w242 w246]
                          frame #0 {
                            n127 = Index Array(array=w242, index=4) -> (element=w241:T6)
                            n128 = call "__move_motor2.vi"("Moving distance"=50.0, "motor setup"=w241) -> ()  [unwired: 2 in, 2 out]
                          }
                          frame #1 {
                            n129 = Index Array(array=w246, index=5) -> (element=w245:T6)
                            n130 = call "__move_motor2.vi"("Moving distance"=50.0, "motor setup"=w245) -> ()  [unwired: 2 in, 2 out]
                          }
                        }
                      }
                    }
                  }
                  frame 2 {
                    n131 = local read "Bias_LO_equip"() -> (w253:T1)
                    n132 = local read "Control"() -> (w252:T2)
                    n133 = Unbundle By Name(w252) -> ("Offset"=w250:dbl, "control"=w251:u16)
                    n134 = call "__SISbias_Set.vi"("SIS　Mode"=w251, "Offset"=w250, "Set_V"=4.0, "Bias_LO_equip"=w253) -> ()  [unwired: 7 in, 1 out]
                  }
                  frame 3 {
                    # "入力をP1に"
                    n135 = local read "Control"() -> (w256:T2)
                    n136 = Unbundle By Name(w256) -> ("6501Dev#"=w255:i16)
                    n137 = call "__SW_8710XB_6501.vi"("Path(1..6)"=2, "ch(1..6)"=5, "bit(4or6)"=4, "Dev(1,2..)"=w255) -> ()
                  }
                }
              }
              frame #5 {
                n138 = Wait (ms)(milliseconds to wait=1000) -> ()  [unwired: 1 out]
              }
              frame #6 {
                n139 = local write "スライド"(2) -> ()
              }
              frame #7 {
                w267 = 2
                # "Cold データ取得"
                n140 = local read "wait"() -> (w273:dbl)
                n141 = Unbundle By Name(w271) -> ("AVEG"=w270:i16)
                n142 = call "__READ_SP_trace_E4440A.vi"("AVG(0-100)"=w270, "wait(s)"=w273, "GPIB"=w274) -> ("error out"=w263:errorcluster, "data"=w272:dbl[])  [unwired: 3 in]
                n143 = Replace Array Subset(array=w269, new element=w272, index (row)=w267) -> (w261:dbl[][])  [unwired: 1 in]
                n144 = Index Array(array=w261, index (row)=0) -> (element=w266:dbl[])  [unwired: 1 in]
                n145 = Index Array(array=w261, index (row)=w267) -> (element=w265:dbl[])  [unwired: 1 in]
                n146 = Unbundle By Name(w263) -> ("status"=w262:bool)
                n147 = Build Cluster Array(w266, w265) -> (w264:cluster{dbl, dbl}[])
                n148 = local write "XYグラフ"(w264) -> ()
              }
              frame #8 {
                n149 = local write "OKボタン"(FALSE) -> ()
                n150 = Wait (ms)(milliseconds to wait=1000) -> ()  [unwired: 1 out]
              }
            }
            n151 = Compound Arithmetic op=AND(w122, w121) -> (w123:bool)
          }
        }
        frame 4 {
          n152 = while {
            tunnel: w281 -> [w289]
            tunnel: w280 -> [w288]
            tunnel: w279 -> [w287]
            tunnel: [w286] -> w278
            tunnel: w277 -> [w282]
            stop <- w285 continue-if-true
            n153 = stacked-sequence {
              seq-local: [_ w298 _] -> [_ _ w344]
              tunnel: w288 -> [_ w300 _]
              tunnel: w289 -> [_ w301 _]
              tunnel: w287 -> [_ w299 _]
              tunnel: [_ _ w344] -> w286
              tunnel: [_ w297 _] -> w284
              tunnel: [_ _ TRUE] -> w283
              tunnel: w282 -> [_ _ _]
              frame #0 {
                n154 = local write "OKボタン"(TRUE) -> ()
                n155 = local write "スライド"(1) -> ()
              }
              frame #1 {
                n156 = local read "sp_data"() -> (w293:T3)
                n157 = local read "Control"() -> (w295:T2)
                n158 = Unbundle By Name(w293) -> ("ATTcal"=w296:bool)
                n159 = Unbundle By Name(w295) -> ("GPIB_SP"=w292:string, "GPIB_ATT"=w294:string)
                n160 = case shown="거짓" w296 {
                  tunnel: w301 -> [w315 _]
                  tunnel: w300 -> [w312 _]
                  tunnel: w299 -> [w310 w318]
                  tunnel: [w308 w316] -> w298
                  tunnel: [w302 w317] -> w297
                  tunnel: w294 -> [_ w321]
                  tunnel: w293 -> [_ w320]
                  tunnel: w292 -> [_ w319]
                  frame False {
                    w307 = 1
                    # "Hotデータ取得"
                    n161 = local read "wait"() -> (w314:dbl)
                    n162 = Unbundle By Name(w312) -> ("AVEG"=w311:i16)
                    n163 = call "__READ_SP_trace_E4440A.vi"("AVG(0-100)"=w311, "wait(s)"=w314, "GPIB"=w315) -> ("error out"=w303:errorcluster, "data"=w313:dbl[])  [unwired: 3 in]
                    n164 = Replace Array Subset(array=w310, new element=w313, index (row)=w307) -> (w308:dbl[][])  [unwired: 1 in]
                    n165 = Index Array(array=w308, index (row)=0) -> (element=w306:dbl[])  [unwired: 1 in]
                    n166 = Unbundle By Name(w303) -> ("status"=w302:bool)
                    n167 = Index Array(array=w308, index (row)=w307) -> (element=w305:dbl[])  [unwired: 1 in]
                    n168 = Build Cluster Array(w306, w305) -> (w304:cluster{dbl, dbl}[])
                    n169 = local write "XYグラフ"(w304) -> ()
                  }
                  frame True {
                    n170 = stacked-sequence {
                      tunnel: w320 -> [w323 _ w327 w340 _]
                      tunnel: [_ _ w330 _ _] -> w317
                      tunnel: [_ _ w329 _ _] -> w316
                      tunnel: w321 -> [w324 _ _ w342 _]
                      tunnel: w319 -> [_ _ w328 _ _]
                      tunnel: w318 -> [_ _ w326 _ _]
                      frame #0 {
                        n171 = Unbundle By Name(w323) -> ("ATT2"=w322:dbl)
                        n172 = call "__AttSet_11713A.vi"("ATT(dB)"=w322, "GPIB"=w324) -> ()  [unwired: 2 in]
                      }
                      frame #1 {
                        n173 = Wait (ms)(milliseconds to wait=1000) -> ()  [unwired: 1 out]
                      }
                      frame #2 {
                        w335 = 3
                        n174 = local read "wait"() -> (w339:dbl)
                        n175 = Unbundle By Name(w327) -> ("SP_set.AVEG"=w337:i16)
                        n176 = call "__READ_SP_trace_E4440A.vi"("AVG(0-100)"=w337, "wait(s)"=w339, "GPIB"=w328) -> ("error out"=w331:errorcluster, "data"=w338:dbl[])  [unwired: 3 in]
                        n177 = Replace Array Subset(array=w326, new element=w338, index (row)=w335) -> (w329:dbl[][])  [unwired: 1 in]
                        n178 = Index Array(array=w329, index (row)=0) -> (element=w334:dbl[])  [unwired: 1 in]
                        n179 = Index Array(array=w329, index (row)=w335) -> (element=w333:dbl[])  [unwired: 1 in]
                        n180 = Unbundle By Name(w331) -> ("status"=w330:bool)
                        n181 = Build Cluster Array(w334, w333) -> (w332:cluster{dbl, dbl}[])
                        n182 = local write "XYグラフ"(w332) -> ()
                      }
                      frame #3 {
                        n183 = Unbundle By Name(w340) -> ("ATT1"=w341:dbl)
                        n184 = call "__AttSet_11713A.vi"("ATT(dB)"=w341, "GPIB"=w342) -> ()  [unwired: 2 in]
                      }
                      frame #4 {
                        n185 = Wait (ms)(milliseconds to wait=1000) -> ()  [unwired: 1 out]
                      }
                    }
                  }
                }
              }
              frame #2 {
                n186 = local write "OKボタン"(FALSE) -> ()
                n187 = Wait (ms)(milliseconds to wait=1000) -> ()  [unwired: 1 out]
              }
            }
            n188 = Compound Arithmetic op=AND(w284, w283) -> (w285:bool)
          }
        }
      }
    }
    frame #4 {
      # "雑音温度の計算"
      n189 = Unbundle By Name(w356) -> ("ATTcal"=w348:bool)
      n190 = Unbundle By Name(w355) -> ("point"=w354:i16)
      n191 = case shown="거짓" w348 {
        tunnel: w356 -> [w363 w392]
        tunnel: w354 -> [w362 w390]
        tunnel: w357 -> [w361 w393]
        tunnel: [w360 w391] -> w350
        tunnel: [w358 w389] -> w352
        frame False {
          n192 = for {
            N: w362 -> [_]
            tunnel: w363 -> [_]
            tunnel: [w371] -> w358 mode=indexing
            tunnel: w361 -> [w370]
            i -> [w367]
            n193 = local read "Control"() -> (w364:T2)
            n194 = Unbundle By Name(w364) -> ("Th"=w374:dbl, "Tc"=w373:dbl)
            n195 = Index Array(array=w370, index (row)=1, index (col)=w367) -> (element=w366:dbl)
            n196 = Index Array(array=w370, index (row)=2, index (col)=w367) -> (element=w365:dbl)
            n197 = xnode "フォーミュラ2"("ph"=w366, "pc"=w365, "th"=w374, "tc"=w373) -> ("結果"=w372:dbl)  [unwired: 1 in, 1 out]
            n198 = To Double Precision Float(number=w372) -> (double precision float=w371:dbl)
          }
          n199 = Replace Array Subset(array=w361, new element=w358, index (row)=4) -> (w360:dbl[][])  [unwired: 1 in]
        }
        frame True {
          n200 = stacked-sequence {
            seq-local: [w398 _] -> [_ w426]
            tunnel: w393 -> [w400 w424]
            tunnel: w392 -> [_ w427]
            tunnel: [_ w423] -> w391
            tunnel: w390 -> [_ w422]
            tunnel: [_ w421] -> w389
            frame #0 {
              n201 = local read "sp_data"() -> (w420:T3)
              n202 = Unbundle By Name(w420) -> ("SNAdatafile ATT1"=w403:path, "SNAdatafile ATT2"=w402:path)
              n203 = call-poly <vilib>:"Read From Spreadsheet File.vi"("delimiter (\\t)"=",", "transpose (no:F)"=TRUE, "file path (dialog if empty)"=w403) -> ("all rows"=w414:dbl[][])  [unwired: 4 in, 4 out]
              n204 = call-poly <vilib>:"Read From Spreadsheet File.vi"("delimiter (\\t)"=",", "transpose (no:F)"=TRUE, "file path (dialog if empty)"=w402) -> ("all rows"=w406:dbl[][])  [unwired: 4 in, 4 out]
              n205 = Index Array(array=w414, index (row)=0) -> (element=w418:dbl[])  [unwired: 1 in]
              n206 = Index Array(array=w400, index (row)=0) -> (element=w399:dbl[])  [unwired: 1 in]
              n207 = Index Array(array=w406, index (row)=0) -> (element=w410:dbl[])  [unwired: 1 in]
              n208 = Multiply(x=w399, y=1000000000.0) -> (x*y=w397:dbl[])
              n209 = Index Array(array=w414, index (row)=1) -> (element=w417:dbl[])  [unwired: 1 in]
              n210 = Index Array(array=w406, index (row)=1) -> (element=w409:dbl[])  [unwired: 1 in]
              n211 = Bundle("all rows"=w418, "all rows"=w417) -> ()  [unwired: 1 in, 1 out]
              n212 = Bundle("all rows"=w410, "all rows"=w409) -> ()  [unwired: 1 in, 1 out]
              n213 = call <vilib>:"Interpolate 1D.vi"("method"=1, "xi"=w397, "X"=w418, "Y"=w417) -> ("yi"=w395:dbl[])  [unwired: 5 in, 2 out]
              n214 = call <vilib>:"Interpolate 1D.vi"("method"=1, "xi"=w397, "X"=w410, "Y"=w409) -> ("yi"=w394:dbl[])  [unwired: 5 in, 2 out]
              n215 = Subtract(x=w395, y=w394) -> (x-y=w398:dbl[])
            }
            frame #1 {
              n216 = for {
                N: w422 -> [_]
                tunnel: [w441] -> w421 mode=indexing
                tunnel: w424 -> [w436]
                tunnel: w427 -> [_]
                tunnel: w426 -> [w432]
                i -> [w431]
                n217 = local read "Control"() -> (w428:T2)
                n218 = Unbundle By Name(w428) -> ("Th"=w434:dbl, "Tc"=w433:dbl)
                n219 = Index Array(array=w436, index (row)=1, index (col)=w431) -> ()  [unwired: 1 out]
                n220 = Index Array(array=w436, index (row)=3, index (col)=w431) -> (element=w435:dbl)
                n221 = Index Array(array=w436, index (row)=2, index (col)=w431) -> (element=w438:dbl)
                n222 = Index Array(array=w432, index=w431) -> (element=w430:dbl)
                n223 = xnode "フォーミュラ3"("pc"=w438, "th"=w434, "tc"=w433, "patt"=w435, "La"=w430) -> ("結果"=w429:dbl)  [unwired: 1 in, 1 out]
                n224 = To Double Precision Float(number=w429) -> (double precision float=w441:dbl)
              }
              n225 = Replace Array Subset(array=w424, new element=w421, index (row)=4) -> (w423:dbl[][])  [unwired: 1 in]
            }
          }
        }
      }
      n226 = Index Array(array=w350, index (row)=0) -> (element=w349:dbl[])  [unwired: 1 in]
      n227 = Build Cluster Array(w349, w352) -> (→"XYグラフ 2":cluster{dbl, dbl}[])
    }
    frame #5 {
      # "データの保存"
      n228 = Unbundle By Name(w459) -> ("SAVE OFF/ON"=w460:bool)
      n229 = case shown="참" w460 {
        tunnel: w459 -> [_ w465]
        tunnel: w458 -> [_ w463]
        frame False {
        }
        frame True {
          n230 = Unbundle By Name(w465) -> ("file_name"=w464:string)
          n231 = local read "Control"() -> (w462:T2)
          n232 = Unbundle By Name(w462) -> ("DATAパス"=w461:path)
          n233 = call "___save_2d_data_with_header.vi"("配列"=w463, "file_name"=w464, "パス"=w461) -> ()  [unwired: 8 in, 1 out]
        }
      }
    }
  }
